vi "UHR-Fleezers Control (fpga) - avogadro 6 - symmetric position FB_raster scan ALEX.vi"() -> ()   [LabVIEW 2014]
doc: "UHR-Fleezers Instrument Control Code (fpga)"
uses:
  <vilib>/Platform/TimedLoop/XDataNode/timing_clust.ctl
  <vilib>/Platform/TimedLoop/XDataNode/nitl_modes.ctl
  <vilib>/Platform/TimedLoop/XDataNode/wakeup.ctl
  <vilib>/rvi/Emulation/niFpgaGetClockAttributes.vi
  <vilib>/rvi/Emulation/niFpgaSctlEmulationGetInTimedLoop.vi
  <vilib>/rvi/Emulation/niFpgaEmulationReportErrorSimple.vi
  <vilib>/rvi/Emulation/niFpgaProcessEmulError.vi
  <vilib>/rvi/eio/common/nirviEmuTemplateMethod_errors.vi
  <vilib>/rvi/interface/RandomDataEmulation/niFpgaRandomDataHandleErrors.vi
  <vilib>/rvi/Emulation/niFpgaCriticalErrorInLSC.vi
  <vilib>/rvi/Emulation/niFpgaEmulationIsFPGAContextNoSignature.vi
  <vilib>/rvi/errors/niFpgaSetErrorForExecOnDevCompSimple.vi
  <vilib>/rvi/eio/common/nirviEmuReportErrorAndStop.vi
  <vilib>/rvi/DataTransferAndStorage/Container/Common/niFpgaContainerGetUniqueNameForEmu.vi
  <vilib>/rvi/FIFO/Fifo_Resource/nirvififoEmulationSetSize.vi
  <vilib>/rvi/FIFO/Fifo_Resource/nirviFifoEmulationQueueMgr.vi
  <instcachedir>/0/nirviFifoEmulationQueueMgr_E5CAEC123FF24DC58D834DCA3CDAA9B5.lvgen/nirviFifoEmulationQueueMgr_E5CAEC123FF24DC58D834DCA3CDAA9B5_001.vi
  <vilib>/rvi/FIFO/Fifo_Resource/nirvififoEmulationDetermineInputValidOut.vi
  <vilib>/rvi/FIFO/Fifo_Resource/nirvififoEmulationCreateLock.vi
  <vilib>/rvi/FIFO/Fifo_Resource/nirvififoEmulationObtainLock.vi
  <vilib>/rvi/FIFO/Fifo_Resource/nirvififoEmulationReleaseLock.vi
  <vilib>/rvi/occurrence/nirviWaitOnOccurrenceBase.vi
  <vilib>/rvi/errors/nirviReportUnexpectedCaseInternalError.vi
  <vilib>/rvi/errors/nirviReportUnexpectedCaseInternalError (U32).vi
  <vilib>/rvi/DataTransferAndStorage/Container/Common/niFpgaContainerExecOnDevCompGetState.vi
  <vilib>/Utility/error.llb/Clear Errors.vi
  <vilib>/eio/EIONode/EIONode.xnode
  <vilib>/eio/EIOMethodNode/EIOMethodNode.xnode
  <vilib>/rvi/DataTransferAndStorage/Container/XNode/niFpgaContainer.xnode
  <vilib>/rvi/interface/RandomDataEmulation/nirviRandomDataFpgaReadWriteTemplate.vi
  <vilib>/rvi/FIFO/Fifo_Resource/nirvififoEmulationWrite.vi
  <vilib>/rvi/FIFO/Fifo_Resource/niFpgaFifoEmulationRefIn.vi
  <vilib>/addons/control/pid/fpga.llb/XNode/niFpgaPID.xnode
  <vilib>/Platform/TimedLoop/XDataNode/XDataNode.xnode
  <vilib>/rvi/FIFO/Fifo_Resource/nirvififoEmulationRead.vi
  <vilib>/Platform/TimedLoop/XDataNode/XDNodeRunTimeDep.lvlib
  <vilib>/rvi/Memory/Memory_Emulation/niFpgaMemoryEmulationRefIn.vi
panel:
  in  "BD 1 Delay (ticks)":u8
  out "lifetime (ticks)":u16
  in  "Lifetime to FIFO":bool
  in  "Tab Control":T1(tab)=enum."MCL trap control"
  in  "Set 3":bool
  in  "Set 2":bool=TRUE
  in  "Set 1":bool=TRUE
  in  "Trap Pos to FIFO":bool
  in  "N of AI1 Int Acq Sets":i16=2 min=1 max=3 step=1
  out "AI Late Counter":u8
  in  "ai count":u16=400
  in  "+ phase":bool
  in  "Phase count adjustment":i16
  out "Relative phase":i16
  in  "AI to FIFO":bool
  out "BD1 Frequency Out 1":u64
  out "BD1 Frequency Out 2":u64
  out "Trap Pos FIFO Timeout":u16
  out "Trap AI FIFO Timeout":u16
  in  "Trap FIFO Set Timeout":i32
  in  "Tab Control 2":T2(tab)
  in  "Multiple trap 3 position offset \nfile":bool
  in  "Piezo offset Y points":u64
  in  "Piezo offset X points":u64
  in  "Piezo offset Xmin":u64
  in  "Piezo Offset Ymin":u64
  in  "Piezo Offset Increment":u64
  out "BD1 amplitude 1 out":u16
  out "BD1 amplitude 2 out":u16
  in  "FB output range":cluster{"output low":i16, "output high":i16}={"output low"=0, "output high"=3000}
  in  "FB Gains":T3={"proportional gain (Kc)"=10, "integral gain (Kc*Ts/Ti)"=5, "derivative gain (Kc*Td/Ts)"=0}
  in  "RF synth green feedback max":i16=4000
  in  "RD":bool=TRUE
  in  "Swap F1 and F2":bool
  in  "Cont. Scan":bool
  in  "Abort scan":bool
  in  "Cycles per step":u64
  in  "Scan BD":bool
  in  "Number of scans":u16
  in  "Scan steps":u64
  in  "Scan freq.  increment":i64
  out "Scanning":bool
  in  "Start scan":bool
  in  "OSK Bd 1":bool
  in  "Reset Bd 1":bool
  in  "PMODE":bool=TRUE
  in  "Number Interlace Cycles":u8=2 min=1 max=3
  in  "Interlace Off Parameters":u8=1 min=1 max=3
  in  "Interlace ON/OFF":bool
  out "DIO Relative phase":i16
  in  "Phase count adjustment (DIO)":i16
  in  "+ phase (DIO)":bool
  out "DIO Late Counter":u8
  in  "DIO count 1 (ticks)":u16=400
  in  "DIO count 2 (ticks)":u16=400
  in  "DIO count 3 (ticks)":u16=400
  out "AI2 Y Sum Set 2":i16
  out "AI2 Y Sum Set 1":i16
  in  "FB Setpoint Set 1":i16 min=0 step=1
  in  "FB Reset Set 1":bool
  in  "FB On/Off Set 1":bool
  in  "FB Reset Set 2":bool
  in  "FB On/Off Set 2":bool
  in  "FB Setpoint Set 2":i16 min=0 step=1
  out "Scan I":u64
  in  "Amp switch delay":u8=5
  in  "RF synth bd controls green":bool
  in  "Phase Trap 2":fxp<+,14,14>
  in  "Phase Trap 1":fxp<+,14,14>
  in  "Phase offset method":u8
  in  "BD 2 Amplitude 1":u16
  in  "BD 1 Amplitude 1":u16
  in  "BD 2 Frequency 1":u64
  in  "BD 1 Frequency 1":u64
  in  "BD 2 Amplitude 2":u16
  in  "BD 1 Amplitude 2":u16
  in  "BD 2 Frequency 2":u64
  in  "BD 1 Frequency 2":u64
  in  "BD 2 Amplitude 3":u16
  in  "BD 1 Amplitude 3":u16
  in  "BD 2 Frequency 3":u64
  in  "BD 1 Frequency 3":u64
  in  "BD 2 Delay (Ticks)":u8 caption="Count(Ticks)"
  in  "Next trap write delay (ticks)":u8 caption="Count(Ticks)"
  out "Random phase generated":fxp<+,14,14>
  in  "RF phase reset before cycles":bool
  in  "Trap 1 osc enable":bool
  in  "N trap osc periods":i16
  in  "Trap osc period (pts)":i16
  in  "Osc traps":bool
  in  "Initiate trap osc":bool
  in  "Ready Write":bool
  in  "Data":i64
  in  "Address 2":u32
  in  "Osc trap cont.":bool
  in  "Trap 2 osc enable":bool
  out "Piezo X out":i16
  out "Piezo Y out":i16
  in  "Piezo Trap ON/Off (AO3)":i16
  in  "Piezo Trap X (AO5)":i16
  in  "Piezo Trap Y (AO4)":i16
  in  "Symmetric force feedback\nand raster scan":bool
  in  "FB Min frequency":u64
  in  "FB Max Frequency":u64
  in  "Dynamic Force FB (Ronen)":bool
  in  "Trap pos. FB Range":T4={"FB2 output low"=-1.0, "FB2 output high"=0.999969482421875}
  in  "Trap Pos. FB Gains":T5={"proportional gain (Kc)"=0.999969482421875, "integral gain (Kc*Ts/Ti)"=0.999969482421875, "derivative gain (Kc*Td/Ts)"=0.0}
  in  "B factor":fxp<+/-,32,16>
  in  "Negate Diff?":bool
  in  "Diff FB Measurement?":bool
  in  "FB Trig Integrate":u32=1
  out "TTrig?":bool
  in  "TTrig Negate Pos":bool=TRUE
  out "Trap Pos FB Int Signal":fxp<+/-,24,9> format="%.18g"
  out "Trap Pos FB Int-Norm Signal":fxp<+/-,16,1> format="%.16g"
  in  "FPGA TTrig Thresh":i64
  in  "FPGA Trap Trig":bool
  out "Trap Pos FB Action":i64
  in  "Trap Pos. FB Offset Factor":i64
  in  "Trap Pos. FB Mult Factor":i64=2
  in  "Trap Pos. FB Reset":bool
  in  "Trap Pos FB Monitor T1 or T2":bool
  in  "AI1 X Scale":u16
  in  "Trap Pos FB Int Count":u16=100
  in  "Trap Pos FB Negate Action":bool
  out "AI1 X Set 2":fxp<+/-,16,1>
  out "AI1 X Set 1":fxp<+/-,16,1>
  in  "Trap Pos. FB SP":fxp<+/-,16,1>
  in  "Force feedback":bool
  out "TTrig Sig":i64
  out "TTrig Fin Thresh":i64
  in  "ScanTrap 3 or Fl-laser":bool
  in  "1D or 2D Scan?":bool
  in  "Abort scan (MCL)":bool
  in  "MCL Scan Axis":bool
  in  "Cont. Scan (MCL)":bool
  out "Scan I (MCL)":u64
  in  "Number of scans (MCL)":u16
  out "Scanning MCL":bool
  in  "Scan steps (MCL)":u64
  in  "Cycles per step (MCL)":u64
  in  "Scan freq.  increment (MCL)":i16
  in  "Start scan (MCL)":bool
  in  "AO2 (X)":i16
  in  "AO1 (Y)":i16
  out "MCL Late Counter":u8
  in  "MCL count":u32=800
  out "MCL Relative Phase":i16
  in  "Phase count adjustment (MCL)":i16
  in  "+ phase (MCL)":bool
  in  "Lifetime events to read blue":u16=100
  in  "Lifetime read blue fifo":bool
  out "lifetime events in fifo":u16
  out "APD2 int gate":bool
  out "APD3 out state":bool
  in  "APD Gate Operating Mode":u8 max=2 step=1
  in  "Invert APD Gate":bool
  in  "APD Gate OFF Count":u16=100
  in  "APD Gate ON Count":u16=300
  out "APD 1 Gate Late Counter":u8
  out "APD 1 Gate Relative Phase":i16
  in  "Phase count adjustment (APD 1 Gate)":i16
  in  "+ phase (APD 1 Gate)":bool
  out "APD 2 Counts 0":u32
  out "APD 2 Counts 1":u32
  out "APD 1 Counts 0":u32
  out "APD 1 Counts 1":u32
  out "APD1 out state":bool
  in  "APD AO scale factor":i16=1
  in  "APD to FIFO":bool
  in  "APD Acq Rate Count":u32=20000000
  out "APD Acq Late Counter":u8
  out "APD Acq Relative Phase":i16
  in  "Phase Count Adjustment (APD Acq)":i16
  in  "+ phase (APD Acq)":bool
  in  "Phase count adjustment (APD 2 Gate)":i16
  out "APD 2 Gate Late Counter":u8
  out "APD 2 Gate Relative Phase":i16
  in  "+ phase (APD 2 Gate)":bool
  out "APD2 out state":bool
  out "APD 3 Counts 0":u32
  out "APD 3 Counts 1":u32
  out "APD 3 Gate Late Counter":u8
  in  "Phase count adjustment (APD 3 Gate)":i16
  out "APD 3 Gate Relative Phase":i16
  in  "+ phase (APD 3 Gate)":bool
  out "APD1 int gate":bool
  out "APD3 int gate":bool
  in  "Lifetime timeout APD1":u16=200
  in  "Laser choice 2":u8=100
  in  "Laser choice 1":u8=100
  in  "Laser choice 0":u8=100
  in  "FL interlace OFF count 2":u16=100
  in  "FL interlace OFF count 1":u16=100
  in  "FL interlace ON count 2":u16=300
  in  "Fl interlace ON count 1":u16=300
  in  "D3 2":i16
  in  "I3 2":i16=5
  in  "P3 2":i16=10
  in  "Green FB Setpoint 2":i16=250 min=0 step=1
  in  "Green FB Reset 2":bool
  in  "D3":i16
  in  "I3":i16=5
  in  "P3":i16=10
  in  "Green Filter Flipper":bool
  in  "Green FB Count":u16=1200
  out "Green Late Counter":u8
  out "Green FB Relative Phase":i16
  in  "Phase count adjustment (Green FB)":i16=10
  in  "+ phase (Green FB)":bool
  out "Green FB Sum":i16
  in  "Green int current ON count adj":u16=150
  in  "Current Out":u16=30000
  in  "Green FB On/Off":bool
  in  "Green FB Setpoint":i16=250 min=0 step=1
  in  "Green FB Reset":bool
  in  "Operating Mode 2":u8=2 max=2 step=1
  in  "Invert GI 2":bool
  in  "Green interlace OFF count 2":u16=900
  in  "Green interlace ON count 2":u16=300
  out "GI Late Counter 2":u8
  out "GI Relative phase 2":i16
  in  "Phase count adjustment (GI) 2":i16=20
  in  "+ phase (GI) 2":bool
  in  "FL interlace OFF count 0":u16=100
  out "GI Relative phase":i16
  in  "Phase count adjustment (GI)":i16
  in  "+ phase (GI)":bool
  in  "FL interlace ON count 0":u16=300
  out "GI Late Counter":u8
  in  "Invert GI":bool
  in  "Operating Mode":u8 max=2 step=1
  out "green FB running":bool
  in  "+ phase (RI)":bool
  out "RI Relative phase":i16
  out "RI Late Counter":u8
  in  "Red interlace ON count":u16=300
  in  "Red interlace OFF count":u16=100
  in  "Invert RI":bool
  in  "Red Laser Operating Mode":u8 max=2 step=1
  in  "Phase count adjustment (RI)":i16
  out "Red FB Intensity":i16
  in  "RI Current Out":u16=30000
  in  "Red FB On/Off":bool
  in  "D4":i16
  in  "I4":i16=5
  in  "P4":i16=10
  in  "Red FB Setpoint":i16=250 min=0 step=1
  in  "Red FB Reset":bool
  in  "RI Operating Mode 2":u8=2 max=2 step=1
  in  "Invert RI 2":bool
  in  "Phase count adjustment (BI AO)":i16=20
  in  "Blue current ON count adj (AO)":u16=150
  in  "BI Current Out":i16=30000
  in  "Blue FB On/Off":bool
  in  "D5":i16
  in  "I5":i16=5
  in  "P5":i16=10
  in  "Blue FB Setpoint":i16=250 min=0 step=1
  in  "Blue FB Reset":bool
  in  "BI Operating Mode (AO)":u8=2 max=2 step=1
  in  "Invert BI (AO)":bool
  in  "Blue OFF count (AO)":u16=900
  in  "Blue ON count (AO)":u16=300
  out "BI Late Counter (AO)":u8
  out "BI Relative phase (AO)":i16
  in  "+ phase (BI AO)":bool
  in  "Phase count adjustment (BI D)":i16
  in  "Blue Laser Operating Mode (D)":u8 max=2 step=1
  in  "Invert BI (D)":bool
  in  "Blue interlace OFF count (D)":u16=100
  in  "Blue interlace ON count (D)":u16=300
  out "Blue Late Counter (D)":u8
  out "BI Relative phase (D)":i16
  in  "+ phase (BI D)":bool
  out "Blue Intensity":i16
  in  "Invert EMCCD Gate":bool
  in  "EMCCD Gate ON count":u16=300
  in  "EMCCD Gate OFF count":u16=100
  out "EMCCD Late counter":u8
  out "EMCCD relative phase":i16
  in  "+ phase (EMCCD Gate)":bool
  in  "EMCCD Gate Operating Mode":u8 max=2 step=1
  in  "Phase Count Adjustment EMCCD Gate":i16
  # "Raster Scan AOD"
  # "1 (X)"
  # "2 (Y)"
  # "IR Intensity Feedback (RF BD 1)"
  # "FB Gains Set 1"
  # "FB output range 1"
  # "IR Intensity Feedback (RF BD 2) -\nonly when using BD 2 for green laser AOM (not trap Y)"
  # "Keep below 4096 (12 bits) to stay within range of RF board. Going over doesn't saturate, it truncates higher bits."
  # "RF phase offset control"
  # "Methods are:\n0 - Default, do nothing at all (no phase offset writes)\n1 - Manual phase adjustment\n2 - Cycle the phase adjustment using the input phase numbers as increment values for each cycle"
  # "False is usual, True is external loop method"
  # "Parameters if using the external RF switching loop"
  # "Parameters if using the usual internal RF switching method"
  # "FB Triggering Excitation Laser"
  # "Trap Pos. FB Gains"
  # "Trap Pos. FB Range"
  # "AO1 (Y)"
  # "2D"
  # "Trap 3"
  # "1D"
  # "AO2 (X)"
  # "Fl Laser"
  # "APD AO for aligning"
  # "Detection Loop"
  # "Green fluorescent laser digital gate interlacing loop"
  # "0 Forced ON\n1 Forced OFF\n2 Interlacing"
  # "ALEX settings:"
  # "Controls for usual IA ME controls green AOM"
  # "Controls for RF synth board controls green AOM"
  # "Green FB Gains"
  # "Red fluorescent laser digital gate interlacing loop"
  # "Detection Loop"
  # "0 Forced ON\n1 Forced OFF\n2 Interlacing"
  # "Analog/FB Control Loop\n(Disabled)"
  # "Digital Control Loop"
  # "Blue laser intensity reading"
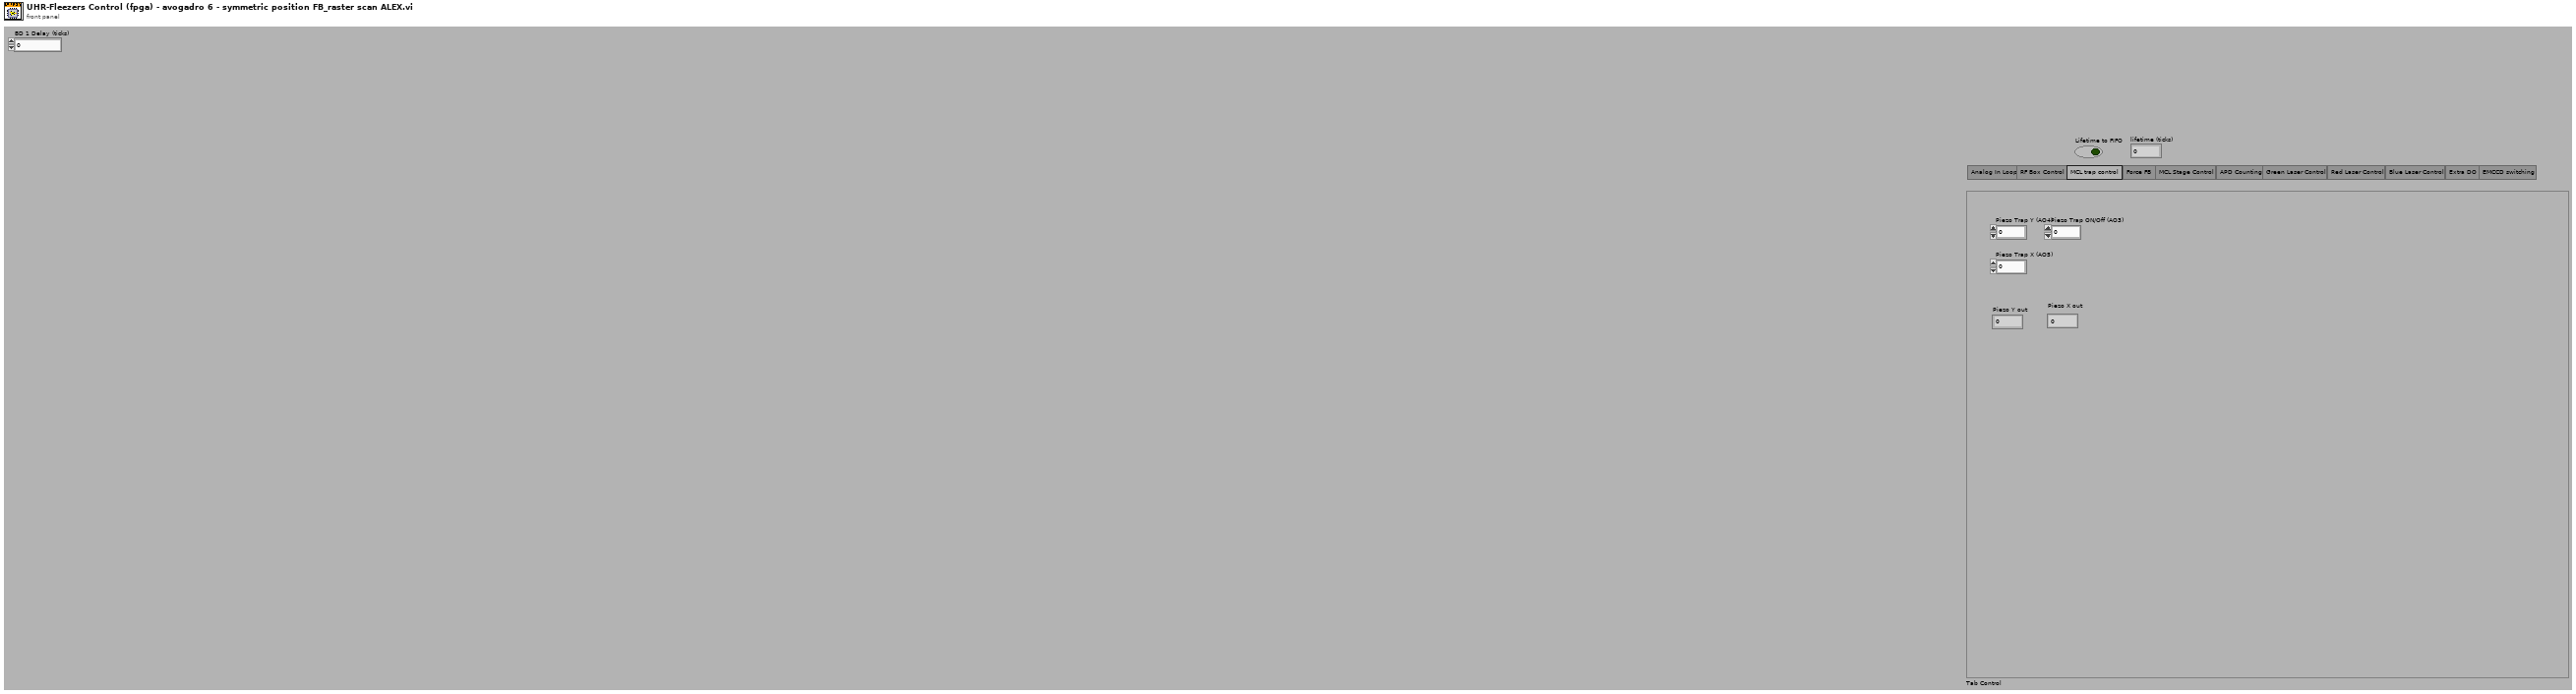
[diagram p1: front panel]
types:
  T1 = enum32{"Analog In Loop", "RF Box Control", "MCL trap control", "Force FB", "MCL Stage Control", "APD Counting", "Green Laser Control", "Red Laser Control", "Blue Laser Control", "Extra DO", "EMCCD switching"}
  T2 = enum32{"Controls", "Interlacing Frequency and Amplitude Values", "Oscillate trap from memory"}
  T3 = cluster{"proportional gain (Kc)":i16, "integral gain (Kc*Ts/Ti)":i16, "derivative gain (Kc*Td/Ts)":i16}
  T4 = cluster{"FB2 output low":fxp<+/-,16,1>, "FB2 output high":fxp<+/-,16,1>}
  T5 = cluster{"proportional gain (Kc)":fxp<+/-,16,1>, "integral gain (Kc*Ts/Ti)":fxp<+/-,16,1>, "derivative gain (Kc*Td/Ts)":fxp<+/-,16,1>}
  T6 = typedef "XDNodeRunTimeDep.lvlib/timing_clust.ctl" = cluster{"Expected End [f-1]":u64, "Actual End [f-1]":u64, "Finished Late? [f-1]":bool, "Expected End [i-1]":u64, "Actual End [i-1]":u64, "Finished Late? [i-1]":bool, "Expected Start [i]":u64, "Actual Start [i]":u64, "Expected Start [f]":u64, "Actual Start [f]":u64, "Source Name":string, "Structure Name":string, "Period":i64, "Deadline":i64, "Offset":i64, "Start":i64, "Priority":i32, "Timeout":i32, "Mode":T7, "Wakeup Reason":T8, "Error":errorcluster, "Source Type":string, "Secondary Source Type":string, "Global End Time":u64, "Global Start Time":u64, "Frame Duration":u64, "Iteration Duration":u64, "Assigned CPU":i32, "I/O Scan Engine Mode":u32}
  T7 = typedef "XDNodeRunTimeDep.lvlib/nitl_modes.ctl" = enum32{"No Change", "Process missed periods, maintain original phase", "Discard missed periods, maintain original phase", "Process missed periods, ignore original phase", "Discard missed periods, ignore original phase"}
  T8 = typedef "XDNodeRunTimeDep.lvlib/wakeup.ctl" = enum32{"Normal", "Aborted", "Asynchronous wakeup", "Timing source error", "Timed loop error", "Timeout"}
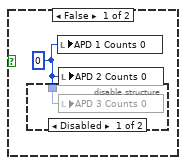
[diagram p4: hidden frame]
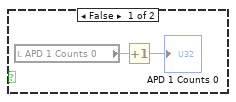
[diagram p9: hidden frame]
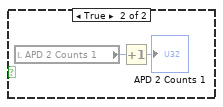
[diagram p11: hidden frame]
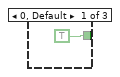
[diagram p13: hidden frame]
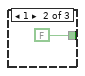
[diagram p14: hidden frame]
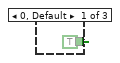
[diagram p15: hidden frame]
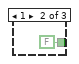
[diagram p16: hidden frame]
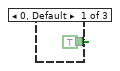
[diagram p18: hidden frame]
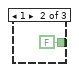
[diagram p19: hidden frame]
diagram:
  w11 = i16 0
  w15 = FALSE
  # "EMCCD gating"
  # "BD2 amp"
  # "BD1 amp"
  # "BD2 amp"
  # "BD1 amp"
  # "timing array current index"
  # "timing array"
  # "timing counter (phase adjusted here)"
  # "late counter"
  n1 = disable-structure shown="Disabled" {
    frame Disabled {
      w16 = i16 2 items=["UnSet Ready", "ReadWrite", "Wait Ready"]
      n2 = while "Handshake memory transfer for trap oscillation sin wave data" {
        shift-right: [w18] -> _
        shift-left: w16 -> [w19]
        stop <- FALSE stop-if-true
        # "Write"
        n3 = case shown="1" w19 {
          tunnel: [w22 w27 w28] -> w18
          frame 3, Default {
            w20 = i16 2 items=["UnSet Ready", "ReadWrite", "Wait Ready"]
            w21 = i16 1 items=["UnSet Ready", "ReadWrite", "Wait Ready"]
            n4 = Select(t=w21, s="Ready Write", f=w20) -> (s? t:f=w22:i16)
          }
          frame 1 {
            w27 = i16 0 items=["UnSet Ready", "ReadWrite", "Wait Ready"]
            n5 = xnode ("Memory Write")("Address"="Address 2", "Data"="Data", "Memory In"=refnum<k21> "Trap osc memory") -> ()  [unwired: 1 out]
          }
          frame 0 {
            w28 = i16 2 items=["UnSet Ready", "ReadWrite", "Wait Ready"]
            n6 = local write "Ready Write"(FALSE ("Ready Read")) -> ()
          }
        }
      }
    }
    frame Enabled {
    }
  }
  n7 = flat-sequence "FPGA initialization to do before running any of the loops" {
    tunnel: [u16 0 ("DIO count 3 (ticks)")] -> w4
    tunnel: [w37] -> _
    frame #0 {
      # "UDCLK out enable and set low"
      # "WR"
      # "BD 2"
      # "BD 1"
      # "With the RF synth board initialization now done in a separate fpga vi, now when this vi is started, board is already configured and is ready for interlacing. Just need to set WR high and enabled UDCLK as write and set to low.\nbefore setting data and address bits."
      # "Start up expansion chassis early\nto avoid delays later"
      # "Set data and address values to something safe (a correct setting) so any initial WR and udclk flipping doesn't have a chance to mess anything up. Safe would be setting an unused data entry:"
      n8 = xnode "FPGA I/O Method Node"("Enable"=TRUE) -> ("FPGA I/O Out"=w31:refnum<k21>)  [unwired: 1 in]
      n9 = xnode "FPGA I/O Method Node"("Enable"=TRUE) -> ("FPGA I/O Out"=w34:refnum<k21>)  [unwired: 1 in]
      n10 = xnode "FPGA I/O Node"("Chassis2/Mod1/AO0"=u16 0 ("Chassis2/Mod4/AO0")) -> ("Chassis2/Mod2/AI0"=w37:i16)  [unwired: 2 in, 2 out]
      n11 = xnode "FPGA I/O Node"("Connector1/DIO15"=TRUE) -> ()  [unwired: 1 in, 1 out]
      n12 = xnode "FPGA I/O Node"("I/O Item"=FALSE ("Connector1/DIO30"), "FPGA I/O In"=w31) -> ()  [unwired: 1 out]
      n13 = xnode "FPGA I/O Node"("I/O Item"=FALSE ("Connector1/DIO30"), "FPGA I/O In"=w34) -> ()  [unwired: 1 out]
      n14 = xnode "FPGA I/O Node"("Connector1/DIO0"=FALSE, "Connector1/DIO1"=FALSE, "Connector1/DIO2"=FALSE, "Connector1/DIO3"=FALSE, "Connector1/DIO4"=FALSE, "Connector1/DIO5"=FALSE, "Connector1/DIO6"=FALSE, "Connector1/DIO7"=FALSE, "Connector1/DIO8"=FALSE, "Connector1/DIO9"=FALSE, "Connector1/DIO10"=FALSE, "Connector1/DIO11"=FALSE, "Connector1/DIO12"=FALSE, "Connector1/DIO13"=FALSE, "Connector1/DIO20"=FALSE, "Connector1/DIO21"=FALSE, "Connector1/DIO22"=FALSE, "Connector1/DIO23"=FALSE, "Connector1/DIO24"=FALSE, "Connector1/DIO25"=FALSE, "Connector1/DIO26"=FALSE, "Connector1/DIO27"=FALSE, "Connector1/DIO14"=FALSE) -> ()  [unwired: 23 in, 23 out]
    }
  }
  n15 = node-c288() -> (w7:T6)  [unwired: 1 in]
  n16 = timed-loop "RF box board DIO control: control bits" {
    timing: w7 -> [_]
    timing-out: [_] -> w6
    tunnel: [w65] -> _
    tunnel: w4 -> [w65]
    stop <- FALSE stop-if-true
    n17 = xnode "FPGA I/O Node"("Connector1/DIO16"="RD", "Connector1/DIO17"="PMODE", "Connector1/DIO18"="OSK Bd 1", "Connector1/DIO19"="Reset Bd 1", "Connector0/DIO3"="Green Filter Flipper") -> ()  [unwired: 5 in, 5 out]
  }
  n18 = node-c288(w6) -> ()
  n19 = local read "AO1 (Y)"() -> (w13:i16)
  n20 = local read "AO2 (X)"() -> (w12:i16)
  n21 = To Unsigned Long Integer(number=w4) -> (unsigned 32bit integer=w3:u32)
  n22 = disable-structure shown="Disabled" {
    disable-tunnel: w4 -> [w73 _]
    disable-tunnel: [w72 _] -> w5
    frame Disabled {
      w72 = FALSE
      n23 = while "APD 1 Gating" {
        shift-right: [w128] -> _
        shift-left: w73 -> [w133]
        shift-right: [w127] -> _
        shift-left: w72 -> [w125]
        stop <- FALSE stop-if-true
        n24 = flat-sequence {
          tunnel: w133 -> [w136]
          tunnel: [w137] -> w131
          tunnel: [w136] -> w129
          tunnel: [w135] -> w126
          tunnel: w125 -> [w135]
          tunnel: [w140] -> w132
          tunnel: w131 -> [w140]
          tunnel: [w139] -> w130
          tunnel: w129 -> [w139]
          tunnel: w126 -> [w138]
          tunnel: [w158] -> w128
          tunnel: w132 -> [w172]
          tunnel: w130 -> [w169]
          tunnel: [w141] -> w127
          frame #0 {
            n25 = call "Loop Timer7"("Count(Ticks)"=w136) -> ("Tick Count(Ticks)"=w137:u16)
          }
          frame #1 {
            # "Signal maybe then sent through \na transistor before APD"
            n26 = xnode "FPGA I/O Node"("Connector0/DIO0"=w138) -> ()  [unwired: 1 in, 1 out]
            "APD1 int gate" <- w138
          }
          frame #2 {
            n27 = feedback #1(TRUE) -> (w164:bool)
            n28 = feedback-in #2(w172) -> ()
            n29 = feedback #2(w172) -> (w171:u16)
            n30 = Not(x=w164) -> (.not. x?=w161:bool)
            n31 = feedback-in #1(w161) -> ()
            n32 = Subtract(x=w172, y=w171) -> (x-y=w170:u16)
            n33 = Select(t="APD Gate ON Count", s=w161, f="APD Gate OFF Count") -> (s? t:f=w166:u16)
            n34 = Subtract(x=w170, y=w169) -> (x-y=w146:u16)
            n35 = Subtract(x=w166, y=w146) -> (x-y=w157:u16)
            n36 = Number To Boolean Array(number=w146) -> (Boolean array=w147:bool[])
            n37 = Or Array Elements(Boolean array=w147) -> (logical OR=w145:bool)
            n38 = Boolean To (0,1)(Boolean="+ phase (APD 1 Gate)") -> (0, 1=w155:i16)
            n39 = Boolean To (0,1)(Boolean=w145) -> (0, 1=w152:i16)
            n40 = Multiply(x=w155, y="Phase count adjustment (APD 1 Gate)") -> (x*y=w153:i16)
            n41 = To Unsigned Byte Integer(number=w152) -> (unsigned 8bit integer=w149:u8)
            n42 = Add(x=w157, y=w153) -> (x+y=w158:u16)
            n43 = feedback #3(i16 0) -> (w160:i16)
            n44 = Subtract(x=w160, y=w153) -> (x-y=w159:i16)
            "APD 1 Gate Relative Phase" <- w159
            n45 = feedback-in #3(w159) -> ()
            n46 = feedback #4(u8 0) -> (w150:u8)
            n47 = Add(x=w149, y=w150) -> (x+y=w148:u8)
            "APD 1 Gate Late Counter" <- w148
            n48 = feedback-in #4(w148) -> ()
            n49 = case shown="2" "APD Gate Operating Mode" {
              tunnel: [TRUE FALSE w175] -> w142
              tunnel: w164 -> [_ _ w175]
              frame 0, Default {
              }
              frame 1 {
              }
              frame 2 {
              }
            }
            n50 = Not(x=w142) -> (.not. x?=w143:bool)
            n51 = Select(t=w143, s="Invert APD Gate", f=w142) -> (s? t:f=w141:bool)
          }
        }
      }
      n52 = while "APD 2 Gating" {
        shift-right: [w77] -> _
        shift-left: w73 -> [w82]
        shift-right: [w76] -> _
        shift-left: w72 -> [w74]
        stop <- FALSE stop-if-true
        n53 = flat-sequence {
          tunnel: w82 -> [w85]
          tunnel: [w86] -> w80
          tunnel: [w85] -> w78
          tunnel: [w84] -> w75
          tunnel: w74 -> [w84]
          tunnel: [w89] -> w81
          tunnel: w80 -> [w89]
          tunnel: [w88] -> w79
          tunnel: w78 -> [w88]
          tunnel: w75 -> [w87]
          tunnel: [w111] -> w77
          tunnel: w81 -> [w121]
          tunnel: w79 -> [w119]
          tunnel: [w90] -> w76
          frame #0 {
            n54 = call "Loop Timer8"("Count(Ticks)"=w85) -> ("Tick Count(Ticks)"=w86:u16)
          }
          frame #1 {
            # "Signal maybe then sent through \na transistor before APD"
            n55 = xnode "FPGA I/O Node"("Connector0/DIO1"=w87) -> ()  [unwired: 1 in, 1 out]
            "APD2 int gate" <- w87
          }
          frame #2 {
            n56 = local read "APD Gate ON Count"() -> (w104:u16)
            n57 = local read "APD Gate OFF Count"() -> (w103:u16)
            n58 = feedback #5(TRUE) -> (w116:bool)
            n59 = feedback-in #6(w121) -> ()
            n60 = feedback #6(w121) -> (w105:u16)
            n61 = Not(x=w116) -> (.not. x?=w114:bool)
            n62 = feedback-in #5(w114) -> ()
            n63 = Subtract(x=w121, y=w105) -> (x-y=w120:u16)
            n64 = Select(t=w104, s=w114, f=w103) -> (s? t:f=w118:u16)
            n65 = Subtract(x=w120, y=w119) -> (x-y=w96:u16)
            n66 = Subtract(x=w118, y=w96) -> (x-y=w110:u16)
            n67 = Number To Boolean Array(number=w96) -> (Boolean array=w95:bool[])
            n68 = Or Array Elements(Boolean array=w95) -> (logical OR=w94:bool)
            n69 = Boolean To (0,1)(Boolean="+ phase (APD 2 Gate)") -> (0, 1=w108:i16)
            n70 = Multiply(x=w108, y="Phase count adjustment (APD 2 Gate)") -> (x*y=w106:i16)
            n71 = Boolean To (0,1)(Boolean=w94) -> (0, 1=w101:i16)
            n72 = Add(x=w110, y=w106) -> (x+y=w111:u16)
            n73 = To Unsigned Byte Integer(number=w101) -> (unsigned 8bit integer=w98:u8)
            n74 = feedback #7(i16 0) -> (w113:i16)
            n75 = Subtract(x=w113, y=w106) -> (x-y=w112:i16)
            "APD 2 Gate Relative Phase" <- w112
            n76 = feedback-in #7(w112) -> ()
            n77 = feedback #8(u8 0) -> (w99:u8)
            n78 = Add(x=w98, y=w99) -> (x+y=w97:u8)
            "APD 2 Gate Late Counter" <- w97
            n79 = feedback-in #8(w97) -> ()
            n80 = local read "APD Gate Operating Mode"() -> (w102:u8)
            n81 = case shown="2" w102 {
              tunnel: [TRUE FALSE w124] -> w91
              tunnel: w116 -> [_ _ w124]
              frame 0, Default {
              }
              frame 1 {
              }
              frame 2 {
              }
            }
            n82 = local read "Invert APD Gate"() -> (w93:bool)
            n83 = Not(x=w91) -> (.not. x?=w92:bool)
            n84 = Select(t=w92, s=w93, f=w91) -> (s? t:f=w90:bool)
          }
        }
      }
    }
    frame Enabled {
    }
  }
  n85 = disable-structure shown="Disabled" {
    disable-tunnel: w4 -> [w176 _]
    frame Disabled {
      n86 = while "Excitation laser intensity feedback measurement (all lasers)" {
        shift-right: [w177] -> _
        shift-left: w176 -> [w182]
        stop <- FALSE stop-if-true
        n87 = flat-sequence {
          tunnel: w182 -> [w184]
          tunnel: [w185] -> w180
          tunnel: [w184] -> w178
          tunnel: [w191] -> w181
          tunnel: w180 -> [w191]
          tunnel: [w190] -> w179
          tunnel: w178 -> [w190]
          tunnel: [w203] -> w177
          tunnel: w181 -> [w214]
          tunnel: w179 -> [w211]
          frame #0 {
            n88 = call "Loop Timer9"("Count(Ticks)"=w184) -> ("Tick Count(Ticks)"=w185:u16)
          }
          frame #1 {
            # "Design note:\n\nAll lasers need to be measured at the same \ntime because the AI expansion module\ncannot independently time the measurements\nwithin our requirements: there is dead time.\n\nThis probably wouldn't be an issue with the built\nin AI on the fpga board itself."
            n89 = xnode "FPGA I/O Node"("Connector1/DIO35"=TRUE) -> ("Chassis2/Mod1/AI2"=→"Blue Intensity", "Chassis2/Mod1/AI1"=→"Red FB Intensity", "Chassis2/Mod1/AI0"=→"Green FB Sum")  [unwired: 4 in, 4 out]
          }
          frame #2 {
            n90 = feedback-in #9(w214) -> ()
            n91 = feedback #9(w214) -> (w213:u16)
            n92 = Subtract(x=w214, y=w213) -> (x-y=w212:u16)
            n93 = xnode "FPGA I/O Node"("Connector1/DIO35"=FALSE) -> ()  [unwired: 1 in, 1 out]
            n94 = Subtract(x=w212, y=w211) -> (x-y=w193:u16)
            n95 = Subtract(x="Green FB Count", y=w193) -> (x-y=w207:u16)
            n96 = Number To Boolean Array(number=w193) -> (Boolean array=w194:bool[])
            n97 = Or Array Elements(Boolean array=w194) -> (logical OR=w192:bool)
            n98 = Boolean To (0,1)(Boolean="+ phase (Green FB)") -> (0, 1=w205:i16)
            n99 = Boolean To (0,1)(Boolean=w192) -> (0, 1=w199:i16)
            n100 = Multiply(x=w205, y="Phase count adjustment (Green FB)") -> (x*y=w200:i16)
            n101 = Add(x=w207, y=w200) -> (x+y=w203:u16)
            n102 = To Unsigned Byte Integer(number=w199) -> (unsigned 8bit integer=w196:u8)
            n103 = feedback #10(i16 0) -> (w202:i16)
            n104 = Subtract(x=w202, y=w200) -> (x-y=w201:i16)
            "Green FB Relative Phase" <- w201
            n105 = feedback-in #10(w201) -> ()
            n106 = feedback #11(u8 0) -> (w197:u8)
            n107 = Add(x=w196, y=w197) -> (x+y=w195:u8)
            "Green Late Counter" <- w195
            n108 = feedback-in #11(w195) -> ()
          }
        }
      }
    }
    frame Enabled {
    }
  }
  n109 = disable-structure shown="Disabled" {
    disable-tunnel: w4 -> [w215 _]
    frame Disabled {
      n110 = while "APD 2 Counter" {
        tunnel: w215 -> [_]
        stop <- FALSE stop-if-true
        n111 = flat-sequence {
          frame #0 {
            n112 = xnode "FPGA I/O Method Node"("FPGA I/O In"=refnum<k21> "Connector0/DIO8" ("APD 2 DO"), "Timeout"=-1) -> ()  [unwired: 2 out]
          }
          frame #1 {
            n113 = local read "APD2 int gate"() -> (w228:bool)
            n114 = case shown="True" w228 {
              frame False {
              }
              frame True {
                n115 = local read "APD2 out state"() -> (w229:bool)
                n116 = case shown="False" w229 {
                  frame False {
                    n117 = local read "APD 2 Counts 0"() -> (w231:u32)
                    n118 = Increment(x=w231) -> (x+1=→"APD 2 Counts 0":u32)
                  }
                  frame True {
                    n119 = local read "APD 2 Counts 1"() -> (w233:u32)
                    n120 = Increment(x=w233) -> (x+1=→"APD 2 Counts 1":u32)
                  }
                }
              }
            }
          }
        }
      }
      n121 = while "APD 1 Counter" {
        tunnel: w215 -> [_]
        stop <- FALSE stop-if-true
        n122 = flat-sequence {
          frame #0 {
            n123 = xnode "FPGA I/O Method Node"("FPGA I/O In"=refnum<k21> "Connector0/DIO4" ("APD 1 DO"), "Timeout"=-1) -> ()  [unwired: 2 out]
          }
          frame #1 {
            n124 = local read "APD1 int gate"() -> (w219:bool)
            n125 = case shown="True" w219 {
              frame False {
              }
              frame True {
                n126 = local read "APD1 out state"() -> (w220:bool)
                n127 = case shown="True" w220 {
                  frame False {
                    n128 = local read "APD 1 Counts 0"() -> (w222:u32)
                    n129 = Increment(x=w222) -> (x+1=→"APD 1 Counts 0":u32)
                  }
                  frame True {
                    n130 = local read "APD 1 Counts 1"() -> (w224:u32)
                    n131 = Increment(x=w224) -> (x+1=→"APD 1 Counts 1":u32)
                  }
                }
              }
            }
          }
        }
      }
    }
    frame Enabled {
    }
  }
  n132 = disable-structure shown="Disabled" {
    disable-tunnel: w4 -> [w234 _]
    frame Disabled {
      w235 = u16 0
      n133 = while "Green and red fluorescent laser interlacing (Current AO to IA 532 nm AOM ME amp)." {
        shift-right: [w315] -> _
        shift-left: w234 -> [w318]
        shift-right: [w312] -> _
        shift-left: w235 -> [w310]
        shift-right: [w309] -> _
        shift-left: w235 -> [w308]
        stop <- FALSE stop-if-true
        n134 = flat-sequence {
          tunnel: w318 -> [w322]
          tunnel: [w323] -> w317
          tunnel: [w322] -> w316
          tunnel: [w321] -> w311
          tunnel: w310 -> [w321]
          tunnel: w308 -> [w320]
          tunnel: [w320] -> w307
          tunnel: [w327] -> w314
          tunnel: w317 -> [w327]
          tunnel: [w326] -> w313
          tunnel: w316 -> [w326]
          tunnel: w311 -> [w325]
          tunnel: w307 -> [w324]
          tunnel: [w355] -> w315
          tunnel: [w371] -> w312
          tunnel: w314 -> [w382]
          tunnel: w313 -> [w379]
          tunnel: [w340] -> w309
          frame #0 {
            n135 = call "Loop Timer10"("Count(Ticks)"=w322) -> ("Tick Count(Ticks)"=w323:u16)
          }
          frame #1 {
            n136 = xnode "FPGA I/O Node"("Chassis2/Mod4/AO0"=w325, "Chassis2/Mod4/AO1"=w324) -> ()  [unwired: 2 in, 2 out]
          }
          frame #2 {
            # "IF RF synth BD does green, never run FB"
            # "ALEX variable is used by APD acquisition loop\nto turn lasers ON/OFF."
            # "Design note:\n\nThese two laser controls are in the same loop\nbecause the expansion current AI cannot separately\ntime the outputs fast enough for us.  Apparently\nit is because of communication time between the\nexpansion card and the fpga.\n\nSo the two analog control signals have the same timing\nand profile, but independent amplitudes to independently\ncontrol the intensity and feedback for each laser."
            n137 = feedback #12(TRUE) -> (w337:bool)
            n138 = Not(x=w337) -> (.not. x?=w338:bool)
            n139 = feedback-in #12(w338) -> ()
            n140 = Subtract(x="Green interlace OFF count 2", y="Green int current ON count adj") -> (x-y=w364:u16)
            n141 = feedback-in #13(w382) -> ()
            n142 = feedback #13(w382) -> (w381:u16)
            n143 = Add(x="Green int current ON count adj", y="Green interlace ON count 2") -> (x+y=w365:u16)
            n144 = Subtract(x=w382, y=w381) -> (x-y=w380:u16)
            n145 = Select(t=w365, s=w338, f=w364) -> (s? t:f=w376:u16)
            n146 = Subtract(x=w380, y=w379) -> (x-y=w348:u16)
            n147 = case shown="2" "RI Operating Mode 2" {
              tunnel: [TRUE FALSE w388] -> w333
              tunnel: w337 -> [_ _ w385]
              frame 0, Default {
              }
              frame 1 {
              }
              frame 2 {
                n148 = Not(x=w385) -> (.not. x?=w387:bool)
                n149 = Select(t=w387, s="Invert RI 2", f=w385) -> (s? t:f=w388:bool)
              }
            }
            n150 = Subtract(x=w376, y=w348) -> (x-y=w359:u16)
            n151 = case shown="2" "Operating Mode 2" {
              tunnel: [TRUE FALSE w422] -> w335
              tunnel: w337 -> [_ _ w419]
              frame 0, Default {
              }
              frame 1 {
              }
              frame 2 {
                n152 = Not(x=w419) -> (.not. x?=w421:bool)
                n153 = Select(t=w421, s="Invert GI 2", f=w419) -> (s? t:f=w422:bool)
              }
            }
            n154 = Number To Boolean Array(number=w348) -> (Boolean array=w349:bool[])
            n155 = Boolean To (0,1)(Boolean="+ phase (GI) 2") -> (0, 1=w361:i16)
            n156 = Or Array Elements(Boolean array=w349) -> (logical OR=w347:bool)
            n157 = local read item#-1() -> (w332)
            n158 = Boolean To (0,1)(Boolean=w347) -> (0, 1=w354:i16)
            n159 = Multiply(x=w361, y="Phase count adjustment (GI) 2") -> (x*y=w357:i16)
            n160 = local read item#-1() -> (w334)
            n161 = local read "RF synth bd controls green"() -> (w329:bool)
            n162 = To Unsigned Byte Integer(number=w354) -> (unsigned 8bit integer=w350:u8)
            n163 = And(x=w332, y=w333) -> (x .and. y?=w331:bool)
            n164 = Add(x=w359, y=w357) -> (x+y=w355:u16)
            n165 = feedback #14(u8 0) -> (w352:u8)
            n166 = Add(x=w350, y=w352) -> (x+y=w351:u8)
            "GI Late Counter 2" <- w351
            n167 = feedback-in #14(w351) -> ()
            n168 = feedback #15(i16 0) -> (w358:i16)
            n169 = Subtract(x=w358, y=w357) -> (x-y=w356:i16)
            "GI Relative phase 2" <- w356
            n170 = feedback-in #15(w356) -> ()
            n171 = And(x=w335, y=w334) -> (x .and. y?=w336:bool)
            n172 = And(x=w336, y="Green FB On/Off") -> (x .and. y?=w366:bool)
            "green FB running" <- w366
            n173 = And(x=w331, y="Red FB On/Off") -> (x .and. y?=w346:bool)
            n174 = Not(x=w329) -> (.not. x?=w328:bool)
            n175 = case shown="True" w346 {
              tunnel: "RI Current Out" -> [w389 _]
              tunnel: [w389 w398] -> w342
              frame False {
              }
              frame True {
                n176 = local read "Red FB Intensity"() -> (w394:i16)
                n177 = Bundle("P4"="P4", "I4"="I4", "D4"="D4") -> (w390:cluster{"P4":i16, "I4":i16, "D4":i16})  [unwired: 1 in]
                n178 = call "Slower PID.vi"("process variable"=w394, "reset?"="Red FB Reset", "setpoint"="Red FB Setpoint", "PID gains (x 2^8)"=w390, "output range"=cluster{"output high":i16, "output low":i16} {"output high"=32767, "output low"=-32768} ("Green FB output range")) -> ("output"=w401:i16)  [unwired: 10 out]
                n179 = To Long Integer(number=w401) -> (32bit integer=w395:i32)
                n180 = Add(x=w395, y=32768) -> (x+y=w397:i32)
                n181 = To Unsigned Word Integer(number=w397) -> (unsigned 16bit integer=w398:u16)
              }
            }
            n182 = And(x=w366, y=w328) -> (x .and. y?=w330:bool)
            n183 = case shown="True" w330 {
              tunnel: "Current Out" -> [w403 w404]
              tunnel: [w403 w404] -> w370
              frame False {
              }
              frame True {
                n184 = disable-structure shown="Disabled" {
                  frame Disabled {
                    n185 = local read "Green FB Sum"() -> (w409:i16)
                    n186 = Bundle("P3"="P3", "I3"="I3", "D3"="D3") -> (w405:cluster{"P3":i16, "I3":i16, "D3":i16})  [unwired: 1 in]
                    n187 = call "Slower PID.vi"("process variable"=w409, "reset?"="Green FB Reset", "setpoint"="Green FB Setpoint", "PID gains (x 2^8)"=w405, "output range"=cluster{"output high":i16, "output low":i16} {"output high"=32767, "output low"=-32768} ("Green FB output range")) -> ("output"=w415:i16)  [unwired: 10 out]
                    n188 = To Long Integer(number=w415) -> (32bit integer=w410:i32)
                    n189 = Add(x=w410, y=32768) -> (x+y=w412:i32)
                    n190 = To Unsigned Word Integer(number=w412) -> ()  [unwired: 1 out]
                  }
                  frame Enabled {
                  }
                }
              }
            }
            n191 = Boolean To (0,1)(Boolean=w331) -> (0, 1=w341:i16)
            n192 = To Unsigned Word Integer(number=w341) -> (unsigned 16bit integer=w343:u16)
            n193 = Boolean To (0,1)(Boolean=w336) -> (0, 1=w372:i16)
            n194 = To Unsigned Word Integer(number=w372) -> (unsigned 16bit integer=w369:u16)
            n195 = Compound Arithmetic op=MULTIPLY(w343, w342) -> (w340:u16)
            n196 = Compound Arithmetic op=MULTIPLY(w369, w370) -> (w371:u16)
          }
        }
      }
      n197 = while "Blue fluorescent laser interlacing (AO control direct to laser)." {
        shift-right: [w242] -> _
        shift-left: w234 -> [w245]
        shift-right: [w239] -> _
        shift-left: i16 0 -> [w237]
        stop <- FALSE stop-if-true
        n198 = flat-sequence {
          tunnel: w245 -> [w248]
          tunnel: [w249] -> w244
          tunnel: [w248] -> w243
          tunnel: [w247] -> w238
          tunnel: w237 -> [w247]
          tunnel: [w252] -> w241
          tunnel: w244 -> [w252]
          tunnel: [w251] -> w240
          tunnel: w243 -> [w251]
          tunnel: w238 -> [w250]
          tunnel: [w262] -> w242
          tunnel: [w278] -> w239
          tunnel: w241 -> [w290]
          tunnel: w240 -> [w287]
          frame #0 {
            n199 = call "Loop Timer13"("Count(Ticks)"=w248) -> ("Tick Count(Ticks)"=w249:u16)
          }
          frame #1 {
            n200 = xnode "FPGA I/O Node"("Connector0/AO3"=w250) -> ()  [unwired: 1 in, 1 out]
          }
          frame #2 {
            n201 = Subtract(x="Blue OFF count (AO)", y="Blue current ON count adj (AO)") -> (x-y=w271:u16)
            n202 = feedback-in #16(w290) -> ()
            n203 = feedback #16(w290) -> (w289:u16)
            n204 = Add(x="Blue current ON count adj (AO)", y="Blue ON count (AO)") -> (x+y=w272:u16)
            n205 = Subtract(x=w290, y=w289) -> (x-y=w288:u16)
            n206 = Subtract(x=w288, y=w287) -> (x-y=w255:u16)
            n207 = Number To Boolean Array(number=w255) -> (Boolean array=w256:bool[])
            n208 = Boolean To (0,1)(Boolean="+ phase (BI AO)") -> (0, 1=w268:i16)
            n209 = Or Array Elements(Boolean array=w256) -> (logical OR=w254:bool)
            n210 = Boolean To (0,1)(Boolean=w254) -> (0, 1=w261:i16)
            n211 = Multiply(x=w268, y="Phase count adjustment (BI AO)") -> (x*y=w264:i16)
            n212 = To Unsigned Byte Integer(number=w261) -> (unsigned 8bit integer=w257:u8)
            n213 = feedback #17(u8 0) -> (w259:u8)
            n214 = Add(x=w257, y=w259) -> (x+y=w258:u8)
            "BI Late Counter (AO)" <- w258
            n215 = feedback-in #17(w258) -> ()
            n216 = feedback #18(i16 0) -> (w265:i16)
            n217 = Subtract(x=w265, y=w264) -> (x-y=w263:i16)
            "BI Relative phase (AO)" <- w263
            n218 = feedback-in #18(w263) -> ()
            n219 = feedback #19(TRUE) -> (w282:bool)
            n220 = case shown="2" "BI Operating Mode (AO)" {
              tunnel: [TRUE FALSE w306] -> w273
              tunnel: w282 -> [_ _ w303]
              frame 0, Default {
              }
              frame 1 {
              }
              frame 2 {
                n221 = Not(x=w303) -> (.not. x?=w305:bool)
                n222 = Select(t=w305, s="Invert BI (AO)", f=w303) -> (s? t:f=w306:bool)
              }
            }
            n223 = And(x=w273, y="Blue FB On/Off") -> (x .and. y?=w274:bool)
            n224 = case shown="True" w274 {
              tunnel: "BI Current Out" -> [w291 _]
              tunnel: [w291 w293] -> w277
              frame False {
              }
              frame True {
                n225 = local read "Blue Intensity"() -> (w292:i16)
                n226 = Bundle("P5"="P5", "I5"="I5", "D5"="D5") -> (w294:cluster{"P5":i16, "I5":i16, "D5":i16})  [unwired: 1 in]
                n227 = call "Slower PID.vi"("process variable"=w292, "reset?"="Blue FB Reset", "setpoint"="Blue FB Setpoint", "PID gains (x 2^8)"=w294, "output range"=cluster{"output high":i16, "output low":i16} {"output high"=32767, "output low"=0} ("Green FB output range")) -> ("output"=w293:i16)  [unwired: 10 out]
              }
            }
            n228 = Not(x=w282) -> (.not. x?=w279:bool)
            n229 = Select(t=w272, s=w279, f=w271) -> (s? t:f=w284:u16)
            n230 = Subtract(x=w284, y=w255) -> (x-y=w266:u16)
            n231 = Add(x=w266, y=w264) -> (x+y=w262:u16)
            n232 = feedback-in #19(w279) -> ()
            n233 = Boolean To (0,1)(Boolean=w273) -> (0, 1=w253:i16)
            n234 = Multiply(x=w253, y=w277) -> (x*y=w278:i16)
          }
        }
      }
    }
    frame Enabled {
    }
  }
  n235 = while "fluorescent laser interlacing (DO)." {
    shift-right: [w429] -> _
    shift-left: w4 -> [w434]
    shift-right: [w428] -> _
    shift-left: w15 -> [w426]
    shift-right: [w425] -> _
    shift-left: u8 0 -> [w423]
    stop <- FALSE stop-if-true
    n236 = flat-sequence {
      tunnel: w434 -> [w438]
      tunnel: [w439] -> w432
      tunnel: [w438] -> w430
      tunnel: [w437] -> w427
      tunnel: w426 -> [w437]
      tunnel: [w436] -> w424
      tunnel: w423 -> [w436]
      tunnel: [w443] -> w433
      tunnel: w432 -> [w443]
      tunnel: [w442] -> w431
      tunnel: w430 -> [w442]
      tunnel: w427 -> [w441]
      tunnel: w424 -> [w440]
      tunnel: [w472] -> w429
      tunnel: w433 -> [w491]
      tunnel: w431 -> [w488]
      tunnel: [w481] -> w428
      tunnel: [w453] -> w425
      frame #0 {
        n237 = call "Loop Timer4"("Count(Ticks)"=w438) -> ("Tick Count(Ticks)"=w439:u16)
      }
      frame #1 {
        n238 = case shown="2" w440 {
          tunnel: w441 -> [w445 w447 w449]
          frame 0, Default {
            w444 = FALSE
            n239 = xnode "FPGA I/O Node"("Connector0/DIO9"=w445, "Connector0/DIO11"=w444, "Connector0/DIO13"=w444) -> ()  [unwired: 3 in, 3 out]
          }
          frame 1 {
            w446 = FALSE
            n240 = xnode "FPGA I/O Node"("Connector0/DIO9"=w446, "Connector0/DIO11"=w447, "Connector0/DIO13"=w446) -> ()  [unwired: 3 in, 3 out]
          }
          frame 2 {
            w448 = FALSE
            n241 = xnode "FPGA I/O Node"("Connector0/DIO9"=w448, "Connector0/DIO11"=w448, "Connector0/DIO13"=w449) -> ()  [unwired: 3 in, 3 out]
          }
        }
      }
      frame #2 {
        # "Laser counting"
        n242 = feedback-in #20(w491) -> ()
        n243 = feedback #20(w491) -> (w490:u16)
        n244 = Subtract(x=w491, y=w490) -> (x-y=w489:u16)
        n245 = Subtract(x=w489, y=w488) -> (x-y=w465:u16)
        n246 = Number To Boolean Array(number=w465) -> (Boolean array=w466:bool[])
        n247 = Or Array Elements(Boolean array=w466) -> (logical OR=w464:bool)
        n248 = feedback #21(u8 0) -> (w462:u8)
        n249 = Increment(x=w462) -> (x+1=w459:u8)
        n250 = Less?(x=u8 5, y=w459) -> (x < y?=w460:bool)
        n251 = Select(t=u8 0, s=w460, f=w459) -> (s? t:f=w451:u8)
        n252 = feedback-in #21(w451) -> ()
        n253 = Boolean To (0,1)(Boolean=w464) -> (0, 1=w471:i16)
        n254 = Quotient & Remainder(x=w451, y=u8 2) -> (floor(x/y)=w450:u8)  [unwired: 1 out]
        n255 = To Unsigned Byte Integer(number=w471) -> (unsigned 8bit integer=w468:u8)
        n256 = feedback #22(u8 0) -> (w469:u8)
        n257 = Add(x=w468, y=w469) -> (x+y=w467:u8)
        "GI Late Counter" <- w467
        n258 = feedback-in #22(w467) -> ()
        n259 = Boolean To (0,1)(Boolean="+ phase (GI)") -> (0, 1=w477:i16)
        n260 = Multiply(x=w477, y="Phase count adjustment (GI)") -> (x*y=w474:i16)
        n261 = feedback #23(i16 0) -> (w475:i16)
        n262 = Subtract(x=w475, y=w474) -> (x-y=w473:i16)
        "GI Relative phase" <- w473
        n263 = feedback-in #23(w473) -> ()
        n264 = feedback #24(TRUE) -> (w484:bool)
        n265 = case shown="2" "Operating Mode" {
          tunnel: [TRUE FALSE w581] -> w481
          tunnel: w484 -> [_ _ w578]
          frame 0, Default {
          }
          frame 1 {
          }
          frame 2 {
            n266 = Not(x=w578) -> (.not. x?=w580:bool)
            n267 = Select(t=w580, s="Invert GI", f=w578) -> (s? t:f=w581:bool)
          }
        }
        n268 = Not(x=w484) -> (.not. x?=w480:bool)
        n269 = case shown="2" w450 {
          tunnel: "FL interlace ON count 0" -> [w501 w528 w555]
          tunnel: "FL interlace OFF count 0" -> [w500 w527 w554]
          tunnel: w480 -> [w499 w526 w557]
          tunnel: [w497 w525 w553] -> w478
          tunnel: w465 -> [w498 w529 w556]
          tunnel: "Fl interlace ON count 1" -> [w496 w524 w552]
          tunnel: "FL interlace OFF count 1" -> [w495 w523 w551]
          tunnel: "FL interlace ON count 2" -> [w494 w522 w550]
          tunnel: "FL interlace OFF count 2" -> [w493 w521 w549]
          tunnel: ["Laser choice 0" "Laser choice 1" "Laser choice 2"] -> w453
          frame 0, Default {
            n270 = case shown="1" "Laser choice 0" {
              tunnel: w501 -> [w506 _ _]
              tunnel: w500 -> [w505 _ _]
              tunnel: w499 -> [w504 w510 w516]
              tunnel: w498 -> [w503 w509 w515]
              tunnel: [w502 w508 w514] -> w497
              tunnel: w496 -> [_ w512 _]
              tunnel: w495 -> [_ w511 _]
              tunnel: w494 -> [_ _ w518]
              tunnel: w493 -> [_ _ w517]
              frame 0, Default {
                n271 = Select(t=w506, s=w504, f=w505) -> (s? t:f=w507:u16)
                n272 = Subtract(x=w507, y=w503) -> (x-y=w502:u16)
              }
              frame 1 {
                n273 = Select(t=w512, s=w510, f=w511) -> (s? t:f=w513:u16)
                n274 = Subtract(x=w513, y=w509) -> (x-y=w508:u16)
              }
              frame 2 {
                n275 = Select(t=w518, s=w516, f=w517) -> (s? t:f=w519:u16)
                n276 = Subtract(x=w519, y=w515) -> (x-y=w514:u16)
              }
            }
          }
          frame 1 {
            n277 = case shown="2" "Laser choice 1" {
              tunnel: w528 -> [w534 _ _]
              tunnel: w527 -> [w533 _ _]
              tunnel: w526 -> [w532 w538 w544]
              tunnel: w529 -> [w531 w537 w543]
              tunnel: [w530 w536 w542] -> w525
              tunnel: w524 -> [_ w540 _]
              tunnel: w523 -> [_ w539 _]
              tunnel: w522 -> [_ _ w546]
              tunnel: w521 -> [_ _ w545]
              frame 0, Default {
                n278 = Select(t=w534, s=w532, f=w533) -> (s? t:f=w535:u16)
                n279 = Subtract(x=w535, y=w531) -> (x-y=w530:u16)
              }
              frame 1 {
                n280 = Select(t=w540, s=w538, f=w539) -> (s? t:f=w541:u16)
                n281 = Subtract(x=w541, y=w537) -> (x-y=w536:u16)
              }
              frame 2 {
                n282 = Select(t=w546, s=w544, f=w545) -> (s? t:f=w547:u16)
                n283 = Subtract(x=w547, y=w543) -> (x-y=w542:u16)
              }
            }
          }
          frame 2 {
            n284 = case shown="2" "Laser choice 2" {
              tunnel: w555 -> [w562 _ _]
              tunnel: w554 -> [w561 _ _]
              tunnel: w557 -> [w560 w566 w572]
              tunnel: w556 -> [w559 w565 w571]
              tunnel: [w558 w564 w570] -> w553
              tunnel: w552 -> [_ w568 _]
              tunnel: w551 -> [_ w567 _]
              tunnel: w550 -> [_ _ w574]
              tunnel: w549 -> [_ _ w573]
              frame 0, Default {
                n285 = Select(t=w562, s=w560, f=w561) -> (s? t:f=w563:u16)
                n286 = Subtract(x=w563, y=w559) -> (x-y=w558:u16)
              }
              frame 1 {
                n287 = Select(t=w568, s=w566, f=w567) -> (s? t:f=w569:u16)
                n288 = Subtract(x=w569, y=w565) -> (x-y=w564:u16)
              }
              frame 2 {
                n289 = Select(t=w574, s=w572, f=w573) -> (s? t:f=w575:u16)
                n290 = Subtract(x=w575, y=w571) -> (x-y=w570:u16)
              }
            }
          }
        }
        n291 = Add(x=w478, y=w474) -> (x+y=w472:u16)
        n292 = feedback-in #24(w480) -> ()
      }
    }
  }
  n293 = while "DAQ AI set 1" {
    shift-right: [w582] -> _
    shift-left: w4 -> [w587]
    stop <- FALSE stop-if-true
    n294 = flat-sequence {
      tunnel: w587 -> [w597]
      tunnel: [w598] -> w585
      tunnel: [w597] -> w584
      tunnel: [w608] -> w595
      tunnel: [w607] -> w594
      tunnel: [w606] -> w593
      tunnel: [w605] -> w592
      tunnel: [w604] -> w591
      tunnel: [w603] -> w590
      tunnel: [w602] -> w589
      tunnel: [w601] -> w588
      tunnel: [w600] -> w586
      tunnel: w585 -> [w600]
      tunnel: w584 -> [w599]
      tunnel: [w599] -> w583
      tunnel: [w640] -> w582
      tunnel: w595 -> [w666]
      tunnel: w594 -> [w632]
      tunnel: w593 -> [w633]
      tunnel: w592 -> [w610]
      tunnel: w591 -> [w656]
      tunnel: w590 -> [w655]
      tunnel: w589 -> [w654]
      tunnel: w588 -> [w653]
      tunnel: w586 -> [w650]
      tunnel: w583 -> [w647]
      frame #0 {
        n295 = call "Loop Timer3"("Count(Ticks)"=w597) -> ("Tick Count(Ticks)"=w598:u16)
      }
      frame #1 {
        # "Signal changed to DIO15 to ease\nmeasurement in the room - change\nback for large code"
        n296 = xnode "FPGA I/O Node"("Connector0/DIO15"=TRUE ("Connector1/DIO33")) -> ("Connector0/AI0"=w608:i16, "Connector0/AI1"=w607:i16, "Connector0/AI2"=w606:i16, "Connector0/AI3"=w605:i16, "Connector0/AI4"=w604:i16, "Connector0/AI5"=w603:i16, "Connector0/AI6"=w602:i16, "Connector0/AI7"=w601:i16)  [unwired: 9 in, 9 out]
      }
      frame #2 {
        w636 = FALSE ("AI to FIFO")
        # "Normalize by trap bead QPD sum, AI3"
        # "Adjust phase after data acquired if button pressed"
        n297 = feedback #25(i16 1) -> (w659:i16)
        n298 = Increment(x=w659) -> (x+1=w665:i16)
        n299 = Scale By Power Of 2(n="AI1 X Scale", x=w632) -> (x*2^n=w630:i16)
        n300 = Greater?(x=w665, y="N of AI1 Int Acq Sets") -> (0:w662:bool)
        n301 = Select(t=i16 1, s=w662, f=w665) -> (s? t:f=w664:i16)
        n302 = feedback-in #25(w664) -> ()
        n303 = Divide(x=w630, y=w610) -> (x/y=w629:fxp<+/-,16,1>)
        n304 = feedback #26(w636) -> (w634:bool)
        n305 = feedback #27(w636) -> (w652:bool)
        n306 = case shown="1, Default" w659 {
          tunnel: w633 -> [w691 w698 _]
          tunnel: ["Set 1" "Set 2" "Set 3"] -> w657
          tunnel: ["AI to FIFO" w700 w705] -> w651
          tunnel: w652 -> [_ w700 w705]
          tunnel: ["Trap Pos to FIFO" w699 w704] -> w635
          tunnel: w634 -> [_ w699 w704]
          tunnel: w629 -> [w690 w697 _]
          tunnel: [w689 w695 FALSE] -> w616
          tunnel: [w688 w696 u64 0 ("BD1 Frequency Out 2")] -> w615
          frame 1, Default {
            n307 = local read "BD1 Frequency Out 1"() -> (w688:u64)
            n308 = Compound Arithmetic op=AND("Trap Pos to FIFO", "Set 1", "AI to FIFO") -> (w689:bool)
            "AI2 Y Sum Set 1" <- w691
            "AI1 X Set 1" <- w690
          }
          frame 2 {
            n309 = local read "BD1 Frequency Out 2"() -> (w696:u64)
            n310 = Compound Arithmetic op=AND(w699, "Set 2", w700) -> (w695:bool)
            "AI2 Y Sum Set 2" <- w698
            "AI1 X Set 2" <- w697
          }
          frame 3 {
          }
        }
        n311 = And(x=w657, y=w651) -> (x .and. y?=w658:bool)
        n312 = case shown="True" w658 {
          tunnel: w666 -> [_ w719]
          tunnel: w632 -> [_ w718]
          tunnel: w633 -> [_ w717]
          tunnel: w610 -> [_ w716]
          tunnel: w656 -> [_ w715]
          tunnel: w655 -> [_ w714]
          tunnel: w654 -> [_ w713]
          tunnel: w653 -> [_ w712]
          tunnel: 0 ("DMA buffer timeout") -> [_ w721]
          frame False {
          }
          frame True {
            n313 = Build Array(w719, w718, w717, w716, w715, w714, w713, w712) -> (w720:i16[])
            n314 = for {
              tunnel: w720 -> [w723] mode=indexing
              tunnel: w721 -> [w724]
              tunnel: [w722] -> w710 mode=indexing
              n315 = xnode ("FIFO Write")("Element"=w723, "Timeout"=w724) -> ("Timed Out?"=w722:bool)  [unwired: 1 in, 1 out]
            }
            n316 = Or Array Elements(Boolean array=w710) -> (logical OR=w707:bool)
            n317 = Boolean To (0,1)(Boolean=w707) -> (0, 1=w709:i16)
            n318 = feedback #28(u16 0) -> (w708:u16)
            n319 = Add(x=w709, y=w708) -> (x+y=w706:u16)
            "Trap AI FIFO Timeout" <- w706
            n320 = feedback-in #28(w706) -> ()
          }
        }
        n321 = feedback-in #26(w635) -> ()
        n322 = feedback-in #27(w651) -> ()
        n323 = local read "Piezo X out"() -> (w612:i16)
        n324 = local read "Piezo Y out"() -> (w611:i16)
        n325 = case shown="True" w616 {
          tunnel: w615 -> [_ w674]
          tunnel: [u8 0 w671] -> w614
          tunnel: w612 -> [_ w670]
          tunnel: w611 -> [_ w669]
          frame False {
          }
          frame True {
            n326 = Split Number(x=w674) -> (hi(x)=w675:u32, lo(x)=w676:u32)
            n327 = Split Number(x=w675) -> (lo(x)=w677:u16)  [unwired: 1 out]
            n328 = Split Number(x=w676) -> (hi(x)=w678:u16, lo(x)=w679:u16)
            n329 = Build Array "BD 1 nu Stack"(w677, w678, w679, w670, w669) -> (w673:u16[])
            n330 = for {
              tunnel: w673 -> [w686] mode=indexing
              shift-right: [w682] -> w671
              shift-left: u8 0 -> [w683]
              n331 = xnode ("FIFO Method Node")("Element"=w686, "Timeout"="Trap FIFO Set Timeout") -> ("Timed Out?"=w685:bool)  [unwired: 1 in, 1 out]
              n332 = Boolean To (0,1)(Boolean=w685) -> (0, 1=w684:i16)
              n333 = To Unsigned Byte Integer(number=w684) -> (unsigned 8bit integer=w681:u8)
              n334 = Add(x=w681, y=w683) -> (x+y=w682:u8)
            }
          }
        }
        n335 = To Unsigned Word Integer(number=w614) -> (unsigned 16bit integer=w613:u16)
        n336 = feedback #29(u16 0) -> (w627:u16)
        n337 = Add(x=w613, y=w627) -> (x+y=w626:u16)
        "Trap Pos FIFO Timeout" <- w626
        n338 = feedback-in #29(w626) -> ()
        n339 = feedback-in #30(w650) -> ()
        n340 = feedback #30(w650) -> (w649:u16)
        n341 = Subtract(x=w650, y=w649) -> (x-y=w648:u16)
        n342 = xnode "FPGA I/O Node"("Connector0/DIO15"=FALSE ("Connector1/DIO34")) -> ()  [unwired: 1 in, 1 out]
        n343 = Subtract(x=w648, y=w647) -> (x-y=w618:u16)
        n344 = Boolean To (0,1)(Boolean="+ phase") -> (0, 1=w643:i16)
        n345 = Multiply(x=w643, y="Phase count adjustment") -> (x*y=w637:i16)
        n346 = Subtract(x="ai count", y=w618) -> (x-y=w641:u16)
        n347 = Number To Boolean Array(number=w618) -> (Boolean array=w619:bool[])
        n348 = feedback #31(i16 0) -> (w639:i16)
        n349 = Add(x=w641, y=w637) -> (x+y=w640:u16)
        n350 = Subtract(x=w639, y=w637) -> (x-y=w638:i16)
        "Relative phase" <- w638
        n351 = feedback-in #31(w638) -> ()
        n352 = Or Array Elements(Boolean array=w619) -> (logical OR=w617:bool)
        n353 = Boolean To (0,1)(Boolean=w617) -> (0, 1=w624:i16)
        n354 = To Unsigned Byte Integer(number=w624) -> (unsigned 8bit integer=w621:u8)
        n355 = feedback #32(u8 0) -> (w622:u8)
        n356 = Add(x=w621, y=w622) -> (x+y=w620:u8)
        "AI Late Counter" <- w620
        n357 = feedback-in #32(w620) -> ()
      }
    }
  }
  n358 = while "MCL stage control" {
    shift-right: [w748] -> _
    shift-left: w4 -> [w751]
    shift-right: [w741] -> _
    shift-left: w13 -> [w738]
    shift-right: [w740] -> _
    shift-left: w12 -> [w736]
    shift-right: [w735] -> _
    shift-left: w11 -> [w730]
    shift-right: [w733] -> _
    shift-left: w11 -> [w725]
    shift-right: [w731] -> _
    shift-left: w11 -> [w727]
    stop <- FALSE stop-if-true
    n359 = flat-sequence {
      tunnel: w751 -> [w758]
      tunnel: [w759] -> w747
      tunnel: [w758] -> w745
      tunnel: [w757] -> w739
      tunnel: w738 -> [w757]
      tunnel: [w756] -> w737
      tunnel: w736 -> [w756]
      tunnel: w730 -> [w755]
      tunnel: [w755] -> w729
      tunnel: [w754] -> w728
      tunnel: w727 -> [w754]
      tunnel: [w753] -> w726
      tunnel: w725 -> [w753]
      tunnel: w747 -> [w766]
      tunnel: [w766] -> w746
      tunnel: w745 -> [w765]
      tunnel: [w765] -> w744
      tunnel: w739 -> [w764]
      tunnel: w737 -> [w763]
      tunnel: w729 -> [w762]
      tunnel: w728 -> [w761]
      tunnel: w726 -> [w760]
      tunnel: w746 -> [w780]
      tunnel: w744 -> [w779]
      tunnel: [w780] -> w750
      tunnel: [w779] -> w749
      tunnel: [w778] -> w743
      tunnel: [w777] -> w742
      tunnel: [w769] -> w734
      tunnel: [w767] -> w732
      tunnel: [w887] -> w748
      tunnel: w750 -> [w894]
      tunnel: w749 -> [w891]
      tunnel: w743 -> [w889]
      tunnel: w742 -> [w888]
      tunnel: [w889] -> w741
      tunnel: [w888] -> w740
      tunnel: [w870] -> w735
      tunnel: w734 -> [w870]
      tunnel: [w869] -> w733
      tunnel: w732 -> [w869]
      tunnel: ["Piezo Trap ON/Off (AO3)"] -> w731
      frame #0 {
        n360 = call "Loop Timer5"("Count(Ticks)"=w758) -> ("Tick Count(Ticks)"=w759:u32)
      }
      frame #1 {
        n361 = xnode "FPGA I/O Node"("Connector0/AO1"=w764, "Connector0/AO2"=w763, "Connector0/AO3"=w761, "Connector0/AO4"=w762, "Connector0/AO5"=w760) -> ()  [unwired: 5 in, 5 out]
      }
      frame #2 {
        n362 = local read "Scanning MCL"() -> (w792:bool)
        n363 = Or(x=w792, y="Start scan (MCL)") -> (x .or. y?=w787:bool)
        n364 = Not(x="Abort scan (MCL)") -> (.not. x?=w785:bool)
        n365 = And(x=w785, y=w787) -> (x .and. y?=w784:bool)
        n366 = case "Raster scan" shown="False" w784 {
          tunnel: [w825 w868] -> w789
          tunnel: "Start scan (MCL)" -> [_ w853]
          tunnel: [w825 w829] -> w773
          frame False {
            w825 = i16 0
            n367 = local write "Scanning MCL"(FALSE ("scanning")) -> ()
          }
          frame True {
            w839 = i16 0
            w838 = u64 0
            # "scan incr."
            # "freq. incr. mult."
            # "count steps"
            # "count number of cycles"
            n368 = feedback #33(w838) -> (w865:u64)
            n369 = Select(t=w838, s=w853, f=w865) -> (s? t:f=w867:u64)
            n370 = Increment(x=w867) -> (x+1=w864:u64)
            n371 = Greater?(x="Cycles per step (MCL)", y=w864) -> (0:w848:bool)
            n372 = Select(t=w864, s=w848, f=w838) -> (s? t:f=w863:u64)
            n373 = feedback-in #33(w863) -> ()
            n374 = feedback #34(w838) -> (w862:u64)
            n375 = Select(t=w838, s=w853, f=w862) -> (s? t:f=w857:u64)
            n376 = Increment(x=w857) -> (x+1=w861:u64)
            n377 = Add(x="Scan steps (MCL)", y="Scan steps (MCL)") -> (x+y=w860:u64)
            n378 = Select(t=w857, s=w848, f=w861) -> (s? t:f=w843:u64)
            n379 = Greater?(x=w860, y=w843) -> (0:w842:bool)
            n380 = Select(t=w843, s=w842, f=w838) -> (s? t:f=w858:u64)
            n381 = feedback-in #34(w858) -> ()
            n382 = Equal?(x="Scan steps (MCL)", y=w843) -> (x = y?=w847:bool)
            n383 = Greater?(x="Scan steps (MCL)", y=w857) -> (0:w856:bool)
            n384 = feedback #35(w839) -> (w859:i16)
            n385 = Select(t=w839, s=w853, f=w859) -> (s? t:f=w845:i16)
            n386 = Increment(x=w845) -> (x+1=w855:i16)
            n387 = Decrement(x=w845) -> (x-1=w854:i16)
            n388 = Select(t=w855, s=w856, f=w854) -> (s? t:f=w846:i16)
            n389 = Select(t=w845, s=w847, f=w846) -> (s? t:f=w844:i16)
            n390 = Select(t=w845, s=w848, f=w844) -> (s? t:f=w840:i16)
            n391 = Select(t=w840, s=w842, f=w839) -> (s? t:f=w841:i16)
            n392 = feedback-in #35(w841) -> ()
            n393 = feedback #36(w838) -> (w852:u64)
            n394 = Select(t=w838, s=w853, f=w852) -> (s? t:f=w827:u64)
            n395 = Increment(x=w827) -> (x+1=w849:u64)
            n396 = Select(t=w827, s=w842, f=w849) -> (s? t:f=w828:u64)
            n397 = Greater?(x="Number of scans (MCL)", y=w828) -> (0:w835:bool)
            n398 = Multiply(x="Scan freq.  increment (MCL)", y=w845) -> (x*y=w868:i16)
            n399 = Select(t=TRUE, s="Cont. Scan (MCL)", f=w835) -> (s? t:f=w834:bool)
            "Scanning MCL" <- w834
            n400 = Select(t=w828, s=w834, f=w838) -> (s? t:f=w850:u64)
            n401 = feedback-in #36(w850) -> ()
            n402 = Increment(x=w828) -> (x+1=→"Scan I (MCL)":u64)
            n403 = To Word Integer(number=w827) -> (16bit integer=w830:i16)
            n404 = Multiply(x=w830, y="Scan freq.  increment (MCL)") -> (x*y=w829:i16)
          }
        }
        n405 = case shown="True" "Multiple trap 3 position offset \nfile" {
          tunnel: ["Piezo Trap Y (AO4)" w812] -> w770
          tunnel: ["Piezo Trap X (AO5)" w811] -> w768
          frame False {
          }
          frame True {
            n406 = local read "Scan I"() -> (w823:u64)
            n407 = Decrement(x=w823) -> (x-1=w824:u64)
            n408 = Quotient & Remainder(x=w824, y="Piezo offset Y points") -> (x-y*floor(x/y)=w821:u64, floor(x/y)=w819:u64)
            n409 = Multiply(x=w821, y="Piezo Offset Increment") -> (x*y=w818:u64)
            n410 = Multiply(x="Piezo Offset Increment", y=w819) -> (x*y=w816:u64)
            n411 = Add(x=w816, y="Piezo offset Xmin") -> (x+y=w813:u64)
            n412 = Add(x=w818, y="Piezo Offset Ymin") -> (x+y=w814:u64)
            n413 = To Word Integer(number=w813) -> (16bit integer=w811:i16)
            n414 = To Word Integer(number=w814) -> (16bit integer=w812:i16)
          }
        }
        n415 = Select(t=w773, s="1D or 2D Scan?", f=i16 0) -> (s? t:f=w774:i16)
        n416 = Select(t=w789, s="MCL Scan Axis", f=w774) -> (s? t:f=w790:i16)
        n417 = Select(t=w774, s="MCL Scan Axis", f=w789) -> (s? t:f=w788:i16)
        n418 = case shown="True" "ScanTrap 3 or Fl-laser" {
          tunnel: w790 -> [w800 w802]
          tunnel: w788 -> [w795 w806]
          tunnel: "AO2 (X)" -> [w796 w807]
          tunnel: "AO1 (Y)" -> [w799 w808]
          tunnel: [w798 w808] -> w778
          tunnel: [w797 w807] -> w777
          tunnel: w770 -> [w794 w803]
          tunnel: [w794 w801] -> w769
          tunnel: w768 -> [w793 w805]
          tunnel: [w793 w804] -> w767
          frame False {
            n419 = Add(x=w796, y=w795) -> (x+y=w797:i16)
            n420 = Add(x=w799, y=w800) -> (x+y=w798:i16)
          }
          frame True {
            n421 = Add(x=w803, y=w802) -> (x+y=w801:i16)
            n422 = Add(x=w805, y=w806) -> (x+y=w804:i16)
          }
        }
      }
      frame #3 {
        n423 = feedback-in #37(w894) -> ()
        n424 = feedback #37(w894) -> (w893:u32)
        n425 = Boolean To (0,1)(Boolean="+ phase (MCL)") -> (0, 1=w885:i16)
        n426 = Subtract(x=w894, y=w893) -> (x-y=w892:u32)
        n427 = Multiply(x=w885, y="Phase count adjustment (MCL)") -> (x*y=w881:i16)
        n428 = Subtract(x=w892, y=w891) -> (x-y=w873:u32)
        n429 = Subtract(x="MCL count", y=w873) -> (x-y=w883:u32)
        n430 = feedback #38(i16 0) -> (w882:i16)
        n431 = Subtract(x=w882, y=w881) -> (x-y=w880:i16)
        "MCL Relative Phase" <- w880
        n432 = feedback-in #38(w880) -> ()
        n433 = Number To Boolean Array(number=w873) -> (Boolean array=w874:bool[])
        n434 = Or Array Elements(Boolean array=w874) -> (logical OR=w872:bool)
        n435 = Boolean To (0,1)(Boolean=w872) -> (0, 1=w879:i16)
        n436 = Add(x=w883, y=w881) -> (x+y=w887:u32)
        n437 = To Unsigned Byte Integer(number=w879) -> (unsigned 8bit integer=w876:u8)
        n438 = feedback #39(u8 0) -> (w877:u8)
        n439 = Add(x=w876, y=w877) -> (x+y=w875:u8)
        "MCL Late Counter" <- w875
        n440 = feedback-in #39(w875) -> ()
        "Piezo Y out" <- w870
        "Piezo X out" <- w869
      }
    }
  }
  n441 = while "Trap RF control, main calculations (raster scanning, intensity and position feedback, phase control etc) with primary timing trigger" {
    shift-right: [w912] -> _
    shift-left: w4 -> [w911]
    shift-right: [w910] -> _
    shift-left: FALSE ("Swap F1 and F2") -> [w909]
    shift-right: [w905] -> _
    shift-left: u16 0 ("BD 1 Amplitude 3") -> [w903]
    shift-right: [w902] -> _
    shift-left: u64 0 -> [w901]
    shift-right: [w900] -> _
    shift-left: u64 0 -> [w898]
    shift-right: [w899] -> _
    shift-left: u64 0 -> [w896]
    stop <- FALSE stop-if-true
    n442 = flat-sequence {
      tunnel: w909 -> [w918]
      tunnel: w911 -> [w916]
      tunnel: [w918] -> w908
      tunnel: [w917] -> w907
      tunnel: [w916] -> w906
      tunnel: [w915] -> w904
      tunnel: w903 -> [w915]
      tunnel: [w914] -> w897
      tunnel: w896 -> [w914]
      tunnel: [w931] -> w912
      tunnel: [w930] -> w910
      tunnel: w908 -> [w929]
      tunnel: w907 -> [w928]
      tunnel: w906 -> [w927]
      tunnel: [w926] -> w905
      tunnel: w904 -> [w925]
      tunnel: [w924] -> w902
      tunnel: w901 -> [w923]
      tunnel: [w922] -> w900
      tunnel: [w921] -> w899
      tunnel: w898 -> [w920]
      tunnel: w897 -> [w919]
      frame #0 {
        n443 = call "Loop Timer"("Count(Ticks)"=w916) -> ("Tick Count(Ticks)"=w917:u16)
      }
      frame #1 {
        n444 = flat-sequence {
          tunnel: w929 -> [w939]
          tunnel: w925 -> [w933]
          tunnel: [w995] -> w931
          tunnel: [w1007] -> w930
          tunnel: w928 -> [w1001]
          tunnel: w927 -> [w998]
          tunnel: [w953] -> w926
          tunnel: [w945] -> w924
          tunnel: w923 -> [w944]
          tunnel: [w943] -> w922
          tunnel: [w942] -> w921
          tunnel: w920 -> [w941]
          tunnel: w919 -> [w940]
          frame #0 {
            w934 = -1 ("Timeout")
            # "Operation when you need a long delay for either X or Y to synchonize AOD light out phase (> ~100 ticks)\nor want shorter trap ON timing. Puts some of the delay timing in parallel with the later computations."
            # "Trigger the external loop by sending the boolean FSK value through a FIFO.\nTiming is precise."
            n445 = Boolean To (0,1)(Boolean=w939) -> (0, 1=w938:i16)
            n446 = To Unsigned Word Integer(number=w938) -> (unsigned 16bit integer=w937:u16)
            n447 = xnode ("FIFO Method Node")("Element"=w937, "Timeout"=w934) -> ("FIFO Out"=w936:refnum<k21>)  [unwired: 1 in, 1 out]
            n448 = xnode ("FIFO Method Node")("Element"=w933, "Timeout"=w934, "FIFO In"=w936) -> ("FIFO Out"=w935:refnum<k21>)  [unwired: 1 out]
            n449 = xnode ("FIFO Method Node")("Element"=i16 0, "Timeout"=w934, "FIFO In"=w935) -> ()  [unwired: 2 out]
          }
          frame #1 {
            # "Just counts, wraps around, 8 bit"
            # "Which trap cycle"
            # "Just flips back and forth."
            # "If interlacing is off, this is which cycle to use."
            # "Keep track of trap cycles (trap 1, 2, 3...)"
            # "This is the prior cycle's on time"
            # "increment timing\nindex, reset to 0 if \nend of matrix"
            # "Reset to begginning (1) when number of cycles reached."
            # "timing index"
            # "build byte stacks for writing data\n(must correspond to addresses array constant)"
            # "Timing housekeeping"
            # "Adjust phase if late\n(maintains constant phase relationship between cycles)"
            n450 = feedback #40(u8 0 ("t")) -> (w1004:u8)
            n451 = Increment(x=w1004) -> (x+1=w1043:u8)
            n452 = Increment(x="Number Interlace Cycles") -> (x+1=w1038:u8)
            n453 = Equal?(x=w1043, y=w1038) -> (x = y?=w1045:bool)
            n454 = Select(t=u8 1, s=w1045, f=w1043) -> (s? t:f=w1003:u8)
            n455 = feedback-in #40(w1003) -> ()
            n456 = Increment(x=w1003) -> (x+1=w1040:u8)
            n457 = Equal?(x=w1040, y=w1038) -> (x = y?=w1041:bool)
            n458 = Select "This cycle"(t=u8 1, s=w1041, f=w1040) -> (s? t:f=w1037:u8)
            n459 = Select(t=w1037, s="Interlace ON/OFF", f="Interlace Off Parameters") -> (s? t:f=w963:u8)
            n460 = feedback-in #41(w1001) -> ()
            n461 = feedback #41(w1001) -> (w1000:u16)
            n462 = Select(t=w1003, s="Interlace ON/OFF", f="Interlace Off Parameters") -> (s? t:f=w1036:u8)
            n463 = Subtract(x=w1001, y=w1000) -> (x-y=w999:u16)
            n464 = Subtract "The error"(x=w999, y=w998) -> (x-y=w982:u16)
            n465 = case shown="1, Default" w1036 {
              tunnel: ["DIO count 1 (ticks)" "DIO count 2 (ticks)" "DIO count 3 (ticks)"] -> w997
              frame 1, Default {
              }
              frame 2 {
              }
              frame 3 {
              }
            }
            n466 = Number To Boolean Array(number=w982) -> (Boolean array=w983:bool[])
            n467 = Or Array Elements(Boolean array=w983) -> (logical OR=w981:bool)
            n468 = Boolean To (0,1)(Boolean=w981) -> (0, 1=w988:i16)
            n469 = To Unsigned Byte Integer(number=w988) -> (unsigned 8bit integer=w985:u8)
            n470 = feedback #42(u8 0) -> (w986:u8)
            n471 = Add(x=w985, y=w986) -> (x+y=w984:u8)
            "DIO Late Counter" <- w984
            n472 = feedback-in #42(w984) -> ()
            n473 = Subtract(x=w997, y=w982) -> (x-y=w996:u16)
            n474 = local read "green FB running"() -> (w970:bool)
            n475 = disable-structure shown="Disabled" {
              disable-tunnel: [w1049 _] -> w980
              disable-tunnel: w963 -> [w1046 _]
              frame Disabled {
                n476 = feedback #43(i64 0 ("y")) -> (w1048:i64)
                n477 = case "Synchronize trap oscillations - always begin/end with trap 1" shown="1, Default" w1046 {
                  tunnel: [w1050 w1051 w1052] -> w1049
                  tunnel: w1048 -> [w1050 w1051 _]
                  frame 2 {
                  }
                  frame 3 {
                  }
                  frame 1, Default {
                    n478 = Or(x="Osc traps", y="Initiate trap osc") -> (x .or. y?=w1054:bool)
                    n479 = case "Trap sine oscillation (or whatever pattern is stored in memory)" shown="True" w1054 {
                      tunnel: [i64 0 ("y") w1058] -> w1052
                      tunnel: "Initiate trap osc" -> [_ w1061]
                      frame False {
                      }
                      frame True {
                        w1065 = u16 0
                        w1063 = -1
                        n480 = local write "Initiate trap osc"(FALSE ("Initiate trap osc")) -> ()
                        n481 = feedback #44(w1065) -> (w1067:u16)
                        n482 = Select(t=w1065, s=w1061, f=w1067) -> (s? t:f=w1066:u16)
                        n483 = Greater Or Equal?(x=w1066, y="Trap osc period (pts)") -> (x >= y?=w1072:bool)
                        n484 = Or(x=w1061, y=w1072) -> (x .or. y?=w1073:bool)
                        n485 = Select(t=u16 0, s=w1073, f=w1066) -> (s? t:f=w1057:u16)
                        n486 = feedback #45(w1063) -> (w1064:i32)
                        n487 = Select(t=w1063, s=w1061, f=w1064) -> (s? t:f=w1062:i32)
                        n488 = Increment(x=w1062) -> (x+1=w1069:i32)
                        n489 = Equal?(x=w1057, y=u16 0) -> (x = y?=w1070:bool)
                        n490 = Increment(x=w1057) -> (x+1=w1077:u16)
                        n491 = feedback-in #44(w1077) -> ()
                        n492 = Select(t=w1069, s=w1070, f=w1062) -> (s? t:f=w1068:i32)
                        n493 = feedback-in #45(w1068) -> ()
                        n494 = case shown="False" "Osc trap cont." {
                          tunnel: w1068 -> [w1081 _]
                          frame False {
                            n495 = Greater Or Equal?(x=w1081, y="N trap osc periods") -> (x >= y?=w1079:bool)
                            n496 = Not(x=w1079) -> (.not. x?=w1078:bool)
                            n497 = local write "Osc traps"(w1078) -> ()
                          }
                          frame True {
                          }
                        }
                        n498 = xnode ("Memory Read")("Address"=w1057, "Memory In"=refnum<k21> "Trap osc memory") -> ("Data"=w1058:i64)  [unwired: 1 out]
                      }
                    }
                  }
                }
                n499 = feedback-in #43(w1049) -> ()
              }
              frame Enabled {
              }
            }
            n500 = And(x=w970, y="RF synth bd controls green") -> (x .and. y?=w969:bool)
            n501 = case shown="1, Default" w963 {
              tunnel: [w1205 w1431 "BD 1 Frequency 3"] -> w1033
              tunnel: [w1252 w1430 w1458] -> w972
              tunnel: [w1202 w1428 "BD 1 Amplitude 3"] -> w953
              tunnel: "FB Gains" -> [w1223 w1437 _]
              tunnel: "FB output range" -> [w1224 w1436 _]
              tunnel: w980 -> [w1221 w1434 _]
              tunnel: "BD 2 Frequency 1" -> [w1218 _ _]
              tunnel: "BD 2 Frequency 2" -> [_ w1430 _]
              tunnel: "BD 2 Frequency 3" -> [_ _ w1458]
              tunnel: w969 -> [_ _ w1457]
              tunnel: [w1205 w1429 w1456] -> w945
              tunnel: w944 -> [w1204 w1429 w1456]
              tunnel: [w1197 u64 0 u64 0] -> w943
              tunnel: [w1198 u64 0 u64 0] -> w942
              tunnel: w941 -> [_ w1424 _]
              tunnel: w940 -> [_ w1423 _]
              frame 1, Default {
                w1238 = fxp<+/-,24,9> 0.0 ("AI1 X Set 2")
                w1232 = u16 0
                w1250 = u64 0 ("f")
                # "#Alex This works with div(Q,R) 2, but I think *2^n is faster, untested"
                # "Changed by RG:\nenables symmetric motion of \ntraps during raster scanning \nand force feedback."
                # "Changed by Ronen - correction \nby PID is now implemented not on \nthe Base BD1 frequency but on the last\nfrequency sent."
                # "Added by Ronen -\nUpper and Lower \nLimits for the FB \ngenerated frequency\nto avoid losing bead \nwhen tether breaks"
                # "Explanation of raster scanning:\n1. Cycles: increment counter by 1 every time interlace cycle returns to trap 1. As long as \n  Cycle per Step is larger than counter, keep incrementing counter and do not change step counter.\n  Once counter is equal to Cycles per step, zero counter and increment step counter.\n2. Steps: Increments up every time cycles counter equals cycles per step. Performs the following:\n- To determine DIRECTION of frequency change:  If ScanstepX2 is EQUAL to step counter (full for-back scan finished)\n   frequency increment is set to zero, AND step counter is set to zero. \n   Otherwise: if no change to step counter (because cycleperstep>cycle counter), then no change to frequency\n   increment. \n   If step counter has changed (cycleperstep=cycle counter), then need to figure out direction of frequency change:\n   if step counter is EQUAL to Scansteps: No change to frequency increment\n   Otherwise: If scan steps > step counter - 1 (forward scan NOT completed): increment frequency by 1\n                       If scan steps equal or smaller than step counter -1 (forward scan completed): increment frequency by -1\n\n3. Scans: Increment scan counter every time step counter equals 2Xscan steps (full for-back scan completed)\n    if number of scans > scan counter: Send TRUE to scanning, continue scan\n    if number of scans = scan counter: Send FALSE to Scanning, Scan finished.\n\n  The wire with the asterik can be used as the index for getting the mirror positions in the offset scan."
                # "This signal integration happens no matter what\nso that correct setpoints can be chosen before \nturning on the FB."
                # "Trap 1"
                n502 = local read "AI1 X Set 2"() -> (w1216:fxp<+/-,16,1>)
                n503 = local read "AI1 X Set 1"() -> (w1235:fxp<+/-,16,1>)
                n504 = local read "Scanning"() -> (w1253:bool)
                n505 = Multiply(x=w1216, y="B factor") -> (x*y=w1214:fxp<+/-,48,17>)
                n506 = Or(x=w1253, y="Start scan") -> (x .or. y?=w1248:bool)
                n507 = case shown="True" "Diff FB Measurement?" {
                  tunnel: w1214 -> [w1278 w1287]
                  tunnel: w1235 -> [w1277 w1288]
                  tunnel: [w1275 w1279] -> w1236
                  frame False {
                    n508 = Select(t=w1277, s="Trap Pos FB Monitor T1 or T2", f=w1278) -> (s? t:f=w1275:fxp<+/-,48,17>)
                  }
                  frame True {
                    n509 = Subtract(x=w1288, y=w1287) -> (x-y=w1280:fxp<+/-,48,17>)
                    n510 = Not(x="Negate Diff?") -> (.not. x?=w1286:bool)
                    n511 = Boolean To (0,1)(Boolean="Negate Diff?") -> (0, 1=w1284:i16)
                    n512 = Boolean To (0,1)(Boolean=w1286) -> (0, 1=w1285:i16)
                    n513 = Negate(x=w1284) -> (-x=w1283:i16)
                    n514 = Add(x=w1283, y=w1285) -> (x+y=w1281:i16)
                    n515 = Multiply(x=w1281, y=w1280) -> (x*y=w1279:fxp<+/-,63,32>)
                  }
                }
                n516 = Not(x="Abort scan") -> (.not. x?=w1246:bool)
                n517 = And(x=w1246, y=w1248) -> (x .and. y?=w1245:bool)
                n518 = case "For raster scanning" shown="False" w1245 {
                  tunnel: [i64 0 w1411] -> w1200
                  tunnel: "Start scan" -> [_ w1396]
                  tunnel: [u64 1 w1373] -> w1217
                  frame False {
                    n519 = local write "Scanning"(FALSE ("scanning")) -> ()
                  }
                  frame True {
                    w1380 = i64 0
                    w1379 = u64 0
                    # "scan incr."
                    # "freq. incr. mult."
                    # "count steps"
                    # "count number of cycles"
                    n520 = feedback #46(w1379) -> (w1408:u64)
                    n521 = Select(t=w1379, s=w1396, f=w1408) -> (s? t:f=w1410:u64)
                    n522 = Increment(x=w1410) -> (x+1=w1407:u64)
                    n523 = Greater?(x="Cycles per step", y=w1407) -> (0:w1389:bool)
                    n524 = Select(t=w1407, s=w1389, f=w1379) -> (s? t:f=w1406:u64)
                    n525 = feedback-in #46(w1406) -> ()
                    n526 = feedback #47(w1379) -> (w1405:u64)
                    n527 = Select(t=w1379, s=w1396, f=w1405) -> (s? t:f=w1400:u64)
                    n528 = Increment(x=w1400) -> (x+1=w1404:u64)
                    n529 = Add(x="Scan steps", y="Scan steps") -> (x+y=w1403:u64)
                    n530 = Select(t=w1400, s=w1389, f=w1404) -> (s? t:f=w1384:u64)
                    n531 = Greater?(x=w1403, y=w1384) -> (0:w1383:bool)
                    n532 = Select(t=w1384, s=w1383, f=w1379) -> (s? t:f=w1401:u64)
                    n533 = feedback-in #47(w1401) -> ()
                    n534 = Equal?(x="Scan steps", y=w1384) -> (x = y?=w1388:bool)
                    n535 = Greater?(x="Scan steps", y=w1400) -> (0:w1399:bool)
                    n536 = feedback #48(w1380) -> (w1402:i64)
                    n537 = Select(t=w1380, s=w1396, f=w1402) -> (s? t:f=w1386:i64)
                    n538 = Increment(x=w1386) -> (x+1=w1398:i64)
                    n539 = Decrement(x=w1386) -> (x-1=w1397:i64)
                    n540 = Select(t=w1398, s=w1399, f=w1397) -> (s? t:f=w1387:i64)
                    n541 = Select(t=w1386, s=w1388, f=w1387) -> (s? t:f=w1385:i64)
                    n542 = Select(t=w1386, s=w1389, f=w1385) -> (s? t:f=w1381:i64)
                    n543 = Select(t=w1381, s=w1383, f=w1380) -> (s? t:f=w1382:i64)
                    n544 = feedback-in #48(w1382) -> ()
                    n545 = feedback #49(w1379) -> (w1395:u64)
                    n546 = Select(t=w1379, s=w1396, f=w1395) -> (s? t:f=w1391:u64)
                    n547 = Increment(x=w1391) -> (x+1=w1392:u64)
                    n548 = Select(t=w1391, s=w1383, f=w1392) -> (s? t:f=w1390:u64)
                    n549 = Greater?(x="Number of scans", y=w1390) -> (0:w1376:bool)
                    n550 = Multiply(x="Scan freq.  increment", y=w1386) -> (x*y=w1411:i64)
                    n551 = Select(t=TRUE, s="Cont. Scan", f=w1376) -> (s? t:f=w1375:bool)
                    "Scanning" <- w1375
                    n552 = Select(t=w1390, s=w1375, f=w1379) -> (s? t:f=w1393:u64)
                    n553 = feedback-in #49(w1393) -> ()
                    n554 = Increment(x=w1390) -> (x+1=w1373:u64)
                  }
                }
                "Scan I" <- w1217
                n555 = feedback #50(w1232) -> (w1231:u16)
                n556 = Increment(x=w1231) -> (x+1=w1233:u16)
                n557 = Greater Or Equal?(x=w1233, y="Trap Pos FB Int Count") -> (x >= y?=w1203:bool)
                n558 = Select(t=w1232, s=w1203, f=w1233) -> (s? t:f=w1234:u16)
                n559 = feedback-in #50(w1234) -> ()
                n560 = feedback #51(w1238) -> (w1237:fxp<+/-,24,9>)
                n561 = Add(x=w1236, y=w1237) -> (x+y=w1230:fxp<+/-,24,9>)
                n562 = case "Trap 1 X intensity feedback" shown="True" "FB On/Off Set 1" {
                  tunnel: "BD 1 Amplitude 1" -> [w1413 _]
                  tunnel: [w1413 w1417] -> w1202
                  tunnel: w1224 -> [_ w1414]
                  tunnel: w1223 -> [_ w1415]
                  frame False {
                  }
                  frame True {
                    n563 = local read "AI2 Y Sum Set 1"() -> (w1418:i16)
                    n564 = call "Slower PID.vi"("process variable"=w1418, "reset?"="FB Reset Set 1", "setpoint"="FB Setpoint Set 1", "PID gains (x 2^8)"=w1415, "output range"=w1414) -> ("output"=w1419:i16)  [unwired: 10 out]
                    n565 = To Unsigned Word Integer(number=w1419) -> (unsigned 16bit integer=w1417:u16)
                  }
                }
                "BD1 amplitude 1 out" <- w1202
                n566 = Select(t=w1238, s=w1203, f=w1230) -> (s? t:f=w1241:fxp<+/-,24,9>)
                n567 = feedback-in #51(w1241) -> ()
                n568 = Divide(x=w1230, y="Trap Pos FB Int Count") -> (x/y=w1225:fxp<+/-,16,1>)
                n569 = feedback #52(fxp<+/-,24,9> 0.0 ("AI1 X Set 2")) -> (w1242:fxp<+/-,24,9>)
                n570 = Select(t=w1230, s=w1203, f=w1242) -> (s? t:f=w1243:fxp<+/-,24,9>)
                "Trap Pos FB Int Signal" <- w1243
                n571 = feedback-in #52(w1243) -> ()
                n572 = feedback #53(fxp<+/-,16,1> 0.0 ("Trap Pos FB Int-Norm Signal")) -> (w1227:fxp<+/-,16,1>)
                n573 = Select(t=w1225, s=w1203, f=w1227) -> (s? t:f=w1226:fxp<+/-,16,1>)
                "Trap Pos FB Int-Norm Signal" <- w1226
                n574 = feedback-in #53(w1226) -> ()
                n575 = case "For position feedback" shown="True" "Force feedback" {
                  tunnel: [i64 0 w1294] -> w1199
                  tunnel: w1225 -> [_ w1291]
                  tunnel: w1203 -> [_ w1290]
                  frame False {
                  }
                  frame True {
                    n576 = feedback #54(i64 0) -> (w1293:i64)
                    n577 = case shown="True" w1290 {
                      tunnel: [w1295 w1299] -> w1294
                      tunnel: w1293 -> [w1295 _]
                      tunnel: w1291 -> [_ w1298]
                      frame False {
                      }
                      frame True {
                        n578 = xnode ("PID")("process variable"=w1298, "reset?"="Trap Pos. FB Reset", "setpoint"="Trap Pos. FB SP", "PID gains"="Trap Pos. FB Gains", "output range"="Trap pos. FB Range") -> ("output"=w1308:fxp<+/-,16,1>)
                        n579 = Negate(x=w1308) -> (-x=w1307:fxp<+/-,17,2>)
                        n580 = Select(t=w1307, s="Trap Pos FB Negate Action", f=w1308) -> (s? t:f=w1304:fxp<+/-,17,2>)
                        n581 = Scale By Power Of 2(n=u32 15, x=u32 1) -> (x*2^n=w1301:u32)
                        n582 = Multiply(x=w1304, y=w1301) -> (x*y=w1300:fxp<+/-,17,17>)
                        n583 = To Quad Integer(1:w1300) -> (0:w1312:i64)
                        "Trap Pos FB Action" <- w1312
                        n584 = Multiply(x=w1312, y="Trap Pos. FB Mult Factor") -> (x*y=w1310:i64)
                        n585 = Add(x=w1310, y="Trap Pos. FB Offset Factor") -> (x+y=w1299:i64)
                        n586 = disable-structure shown="Disabled" {
                          disable-tunnel: w1299 -> [w1319 _]
                          frame Disabled {
                            w1323 = u32 0
                            n587 = feedback #55() -> (w1320:i64)  [unwired: 1 in]
                            n588 = Add(x=w1319, y=w1320) -> (x+y=w1317:i64)
                            n589 = feedback #56(w1323) -> (w1325:u32)
                            n590 = Increment(x=w1325) -> (x+1=w1314:u32)
                            n591 = Greater Or Equal?(x=w1314, y="FB Trig Integrate") -> (x >= y?=w1315:bool)
                            n592 = Select(t=i64 0, s=w1315, f=w1317) -> (s? t:f=w1321:i64)
                            n593 = feedback-in #55(w1321) -> ()
                            n594 = Select(t=w1323, s=w1315, f=w1314) -> (s? t:f=w1324:u32)
                            n595 = feedback-in #56(w1324) -> ()
                            n596 = And(x=w1315, y="FPGA Trap Trig") -> (x .and. y?=w1322:bool)
                            n597 = case "Trap FB trigger excitation laser ON" shown="True" w1322 {
                              tunnel: w1317 -> [_ w1329]
                              tunnel: w1314 -> [_ w1327]
                              frame False {
                              }
                              frame True {
                                n598 = Not(x="TTrig Negate Pos") -> (.not. x?=w1336:bool)
                                n599 = Boolean To (0,1)(Boolean="TTrig Negate Pos") -> (0, 1=w1334:i16)
                                n600 = Boolean To (0,1)(Boolean=w1336) -> (0, 1=w1335:i16)
                                n601 = Negate(x=w1334) -> (-x=w1333:i16)
                                n602 = Add(x=w1333, y=w1335) -> (x+y=w1332:i16)
                                n603 = Multiply(x=w1332, y=w1329) -> (x*y=w1331:i64)
                                "TTrig Sig" <- w1331
                                n604 = Multiply(x="FPGA TTrig Thresh", y=w1327) -> (x*y=w1328:i64)
                                "TTrig Fin Thresh" <- w1328
                                n605 = Greater Or Equal?(x=w1331, y=w1328) -> (x >= y?=w1330:bool)
                                n606 = case shown="True" w1330 {
                                frame False {
                                }
                                frame True {
                                w1339 = TRUE ("Green FB On/Off")
                                w1341 = u8 2 ("Operating Mode")
                                n607 = local write "Operating Mode 2"(w1341) -> ()
                                n608 = local write "Operating Mode"(w1341) -> ()
                                n609 = local write "Green FB On/Off"(w1339) -> ()
                                n610 = local write "FPGA Trap Trig"(FALSE ("FPGA Trap Trig")) -> ()
                                "TTrig?" <- w1339
                                }
                                }
                              }
                            }
                          }
                          frame Enabled {
                          }
                        }
                      }
                    }
                    n611 = feedback-in #54(w1294) -> ()
                  }
                }
                n612 = case shown="True" "Symmetric force feedback\nand raster scan" {
                  tunnel: [w1257 w1260] -> w1197
                  tunnel: w1200 -> [w1257 w1261]
                  tunnel: [w1256 w1258] -> w1198
                  tunnel: w1199 -> [w1256 w1259]
                  frame False {
                  }
                  frame True {
                    n613 = Scale By Power Of 2(n=i16 -1, x=w1261) -> (x*2^n=w1260:i64)
                    n614 = Scale By Power Of 2(n=i16 -1, x=w1259) -> (x*2^n=w1258:i64)
                  }
                }
                n615 = And(x="Force feedback", y="Dynamic Force FB (Ronen)") -> (x .and. y?=w1211:bool)
                n616 = case shown="False" w1211 {
                  tunnel: w1198 -> [w1266 w1270]
                  tunnel: [w1265 w1269] -> w1210
                  tunnel: w1204 -> [_ w1268]
                  tunnel: w1203 -> [_ w1267]
                  frame False {
                    # "(BD1 Frequency 1)"
                    n617 = Add(x="BD 1 Frequency 1", y=w1266) -> (x+y=w1265:u64)
                  }
                  frame True {
                    n618 = case shown="True" w1267 {
                      tunnel: w1270 -> [_ w1274]
                      tunnel: [w1271 w1273] -> w1269
                      tunnel: w1268 -> [w1271 w1272]
                      frame False {
                      }
                      frame True {
                        n619 = Add(x=w1272, y=w1274) -> (x+y=w1273:u64)
                      }
                    }
                  }
                }
                n620 = Select(t=w1221, s="Trap 1 osc enable", f=i64 0) -> (s? t:f=w1219:i64)
                n621 = Select(t=w1250, s="Scan BD", f=w1197) -> (s? t:f=w1249:u64)
                n622 = Select(t=w1197, s="Scan BD", f=w1250) -> (s? t:f=w1209:u64)
                n623 = Add(x=w1249, y=w1218) -> (x+y=w1252:u64)
                n624 = Compound Arithmetic op=ADD(w1219, w1210, w1209) -> (w1208:u64)
                n625 = In Range and Coerce(upper limit="FB Max Frequency", x=w1208, lower limit="FB Min frequency") -> (coerced(x)=w1205:u64)  [unwired: 1 out]
                "BD1 Frequency Out 1" <- w1205
              }
              frame 2 {
                # "Trap 2"
                n626 = local read "Symmetric force feedback\nand raster scan"() -> (w1427:bool)
                n627 = case shown="True" w1427 {
                  tunnel: "BD 1 Frequency 2" -> [w1440 w1445]
                  tunnel: [w1440 w1441] -> w1425
                  tunnel: w1424 -> [_ w1444]
                  tunnel: w1423 -> [_ w1442]
                  frame False {
                  }
                  frame True {
                    n628 = Subtract(x=w1445, y=w1444) -> (x-y=w1443:u64)
                    n629 = Subtract(x=w1443, y=w1442) -> (x-y=w1441:u64)
                  }
                }
                n630 = case "Trap 2 X intensity feedback" shown="True" "FB On/Off Set 2" {
                  tunnel: [w1446 w1449] -> w1428
                  tunnel: "BD 1 Amplitude 2" -> [w1446 _]
                  tunnel: w1437 -> [_ w1448]
                  tunnel: w1436 -> [_ w1447]
                  frame False {
                  }
                  frame True {
                    n631 = local read "AI2 Y Sum Set 2"() -> (w1452:i16)
                    n632 = call "Slower PID.vi"("process variable"=w1452, "reset?"="FB Reset Set 2", "setpoint"="FB Setpoint Set 2", "PID gains (x 2^8)"=w1448, "output range"=w1447) -> ("output"=w1450:i16)  [unwired: 10 out]
                    n633 = To Unsigned Word Integer(number=w1450) -> (unsigned 16bit integer=w1449:u16)
                  }
                }
                "BD1 amplitude 2 out" <- w1428
                n634 = Select(t=w1434, s="Trap 2 osc enable", f=i64 0) -> (s? t:f=w1433:i64)
                n635 = Add(x=w1425, y=w1433) -> (x+y=w1431:u64)
                "BD1 Frequency Out 2" <- w1431
              }
              frame 3 {
                # "Fluorescence period"
                n636 = disable-structure shown="Disabled" {
                  disable-tunnel: [w1466 _] -> _
                  disable-tunnel: w1457 -> [w1465 _]
                  frame Disabled {
                    # "Remember if FB was previously on/off"
                    n637 = feedback #57(FALSE) -> (w1461:bool)
                    n638 = case shown="True" w1465 {
                      tunnel: [w1468 w1484] -> w1466
                      tunnel: "BD 2 Amplitude 3" -> [w1468 _]
                      tunnel: [FALSE TRUE] -> w1462
                      tunnel: w1461 -> [_ w1469]
                      frame False {
                      }
                      frame True {
                        # "Makes it so first time FB run when turned on, the PID sees the detector intensity from the last time FB was running, rather than something near zero. Especially assuming the setpoint is not changing, this will make the FB more stable when resuming, and not overshoot the turnon intensity."
                        # "FB output range: 0 should be low, full scale is 12 bits.\nBut be careful not to go over, then higher bits just get ignored by RF board, so output will actually jump down and be unstable. Keep it under 4000 to be safe."
                        n639 = local read "Green FB Sum"() -> (w1472:i16)
                        n640 = feedback-in #58(w1472) -> ()
                        n641 = feedback #58(i16 0 ("Green FB Sum")) -> (w1471:i16)
                        n642 = Select(t=w1472, s=w1469, f=w1471) -> (s? t:f=w1470:i16)
                        n643 = Bundle("P3 2"="P3 2", "I3 2"="I3 2", "D3 2"="D3 2") -> (w1483:cluster{"P3 2":i16, "I3 2":i16, "D3 2":i16})  [unwired: 1 in]
                        n644 = Bundle("RF synth green feedback max"="RF synth green feedback max", i16 0) -> (w1475:cluster{"RF synth green feedback max":i16, i16})  [unwired: 1 in]
                        n645 = call "Slower PID.vi"("process variable"=w1470, "reset?"="Green FB Reset 2", "setpoint"="Green FB Setpoint 2", "PID gains (x 2^8)"=w1483, "output range"=w1475) -> ("output"=w1485:i16)  [unwired: 10 out]
                        n646 = To Unsigned Word Integer(number=w1485) -> (unsigned 16bit integer=w1484:u16)
                      }
                    }
                    n647 = feedback-in #57(w1462) -> ()
                  }
                  frame Enabled {
                  }
                }
              }
            }
            n648 = Split Number(x=w1033) -> (hi(x)=w1032:u32, lo(x)=w1031:u32)
            n649 = Boolean To (0,1)(Boolean="+ phase (DIO)") -> (0, 1=w993:i16)
            n650 = Split Number(x=w1032) -> (lo(x)=w1030:u16)  [unwired: 1 out]
            n651 = Split Number(x=w1031) -> (hi(x)=w1029:u16, lo(x)=w1028:u16)
            n652 = Split Number(x=w1030) -> (hi(x)=w1022:u8, lo(x)=w1021:u8)
            n653 = Split Number(x=w1029) -> (hi(x)=w1020:u8, lo(x)=w1019:u8)
            n654 = Split Number(x=w1028) -> (hi(x)=w1018:u8, lo(x)=w1017:u8)
            n655 = Multiply(x=w993, y="Phase count adjustment (DIO)") -> (x*y=w989:i16)
            n656 = feedback #59(TRUE) -> (w978:bool)
            n657 = Not(x=w978) -> (.not. x?=w977:bool)
            n658 = feedback-in #59(w977) -> ()
            n659 = feedback #60(i16 0) -> (w991:i16)
            n660 = Subtract(x=w991, y=w989) -> (x-y=w990:i16)
            "DIO Relative phase" <- w990
            n661 = feedback-in #60(w990) -> ()
            n662 = Add(x=w996, y=w989) -> (x+y=w995:u16)
            n663 = Build Array "BD 1 nu Stack"(w1022, w1021, w1020, w1019, w1018, w1017) -> (w1016:u8[])
            n664 = case "Store in RF board F1 or F2" shown="True" w977 {
              tunnel: [w1188 w1192] -> w1007
              tunnel: [u8 10 u8 4] -> w1008
              tunnel: "Swap F1 and F2" -> [w1189 w1192]
              tunnel: "BD 2 Frequency 1" -> [_ w1191]
              tunnel: "BD 2 Frequency 2" -> [w1187 _]
              tunnel: [w1187 w1191] -> w973
              frame False {
                # "for RF synth controls\ngreen: F1/F2 stay same"
                # "F2 address (hex)"
                n665 = Not(x=w1189) -> (.not. x?=w1188:bool)
              }
              frame True {
                # "low chooses F1"
                # "F1 address (hex)"
              }
            }
            n666 = Select(t=w973, s="RF synth bd controls green", f=w972) -> (s? t:f=w971:u64)
            n667 = Split Number(x=w971) -> (hi(x)=w1027:u32, lo(x)=w1026:u32)
            n668 = Split Number(x=w1027) -> (lo(x)=w1025:u16)  [unwired: 1 out]
            n669 = Split Number(x=w1026) -> (hi(x)=w1024:u16, lo(x)=w1023:u16)
            n670 = Split Number(x=w1025) -> (hi(x)=w1015:u8, lo(x)=w1014:u8)
            n671 = Split Number(x=w1024) -> (hi(x)=w1013:u8, lo(x)=w1012:u8)
            n672 = Split Number(x=w1023) -> (hi(x)=w1011:u8, lo(x)=w1010:u8)
            n673 = Build Array "BD 2 nu Stack"(w1015, w1014, w1013, w1012, w1011, w1010) -> (w1009:u8[])
            n674 = flat-sequence "Update trap RF synth board settings to be used for the upcoming trap cycle." {
              tunnel: w1009 -> [w1136]
              tunnel: w1016 -> [w1137]
              tunnel: [w1137] -> w967
              tunnel: [w1136] -> w966
              tunnel: w1008 -> [w1138]
              tunnel: w967 -> [w1140]
              tunnel: w966 -> [w1139]
              tunnel: w954 -> [w1151]
              tunnel: w956 -> [w1150]
              tunnel: w955 -> [w1149]
              frame #0 {
                # "To possibly delay\nthese writes to very\nend of loop (for x and\ny phase adjust)"
                n675 = call "Wait8"("Count(Ticks)"="Next trap write delay (ticks)") -> ()  [unwired: 1 out]
              }
              frame #1 {
                # "Next trap RF frequency:\n\nWrite next trap cycle frequency to buffer."
                n676 = for {
                  tunnel: w1140 -> [w1146] mode=indexing
                  tunnel: w1139 -> [w1145] mode=indexing
                  tunnel: w1138 -> [w1143]
                  i -> [w1144]
                  n677 = To Unsigned Byte Integer(number=w1144) -> (unsigned 8bit integer=w1141:u8)
                  n678 = Add(x=w1143, y=w1141) -> (x+y=w1142:u8)
                  n679 = call "write to RF synth bd.vi"("Address Byte"=w1142, "BD 2 Byte"=w1145, "BD 1 Byte"=w1146) -> ()
                }
              }
              frame #2 {
                w1147 = TRUE ("Connector1/DIO15")
                # "Send udclk high\n(BD 1 and 2) to make the new frequency active in F1 or F2 word. But it won't actually be the used frequency until FSK switches to it (begining of next cycle)."
                n680 = xnode "FPGA I/O Node"("Connector1/DIO30"=w1147, "Connector1/DIO29"=w1147) -> ()  [unwired: 2 in, 2 out]
              }
              frame #3 {
                w1148 = FALSE ("Connector1/DIO15")
                n681 = xnode "FPGA I/O Node"("Connector1/DIO30"=w1148, "Connector1/DIO29"=w1148) -> ()  [unwired: 2 in, 2 out]
              }
              frame #4 {
                # "Next trap RF phase offset:\n\nSet the next trap cycle amplitude to the buffer. Won't become active until udclk is set high at proper time at the begining of the next cycle."
                n682 = case shown="True" w1151 {
                  tunnel: w1150 -> [_ w1152]
                  tunnel: w1149 -> [_ w1153]
                  frame False {
                  }
                  frame True {
                    # "phase 1 address start"
                    n683 = for {
                      tunnel: w1152 -> [w1160] mode=indexing
                      tunnel: w1153 -> [w1159] mode=indexing
                      tunnel: u8 0 -> [w1157]
                      i -> [w1158]
                      n684 = To Unsigned Byte Integer(number=w1158) -> (unsigned 8bit integer=w1155:u8)
                      n685 = Add(x=w1157, y=w1155) -> (x+y=w1156:u8)
                      n686 = call "write to RF synth bd.vi"("Address Byte"=w1156, "BD 2 Byte"=w1159, "BD 1 Byte"=w1160) -> ()
                    }
                  }
                }
              }
              frame #5 {
                # "Prep to reset RF phase to zero at start of next cycle. Only reset BD 1. Do nothing to BD 2. This puts the settings in the buffer. A udclk high will make both this phase reset and possibly a new phase offset setting active."
                n687 = case shown="True" "RF phase reset before cycles" {
                  frame False {
                  }
                  frame True {
                    w1163 = u8 66  # BD 1 reset
                    n688 = call "write to RF synth bd.vi"("Address Byte"=u8 31, "BD 2 Byte"=u8 2, "BD 1 Byte"=w1163) -> ()
                  }
                }
              }
              frame #6 {
                # "Address"
                # "Data BD 2"
                # "Data BD 1"
                # "If phase reset wasn't chosen previously, these actions will have no affect. For both BD's, data should be binary 10, and address should be hex 1F (bin 01 1111)"
                # "This sets up the digital communication lines to restart phase accumulation (start RF running agin). It cancels out the possible phase reset. Just need to set WR DIO low then udclk DIOhigh  to make this happen. Doing this here early (and not using the usual board write function) speeds things up.\n\nRestarts RF (BD 1 only, BD2 never stopped in first place)."
                n689 = xnode "FPGA I/O Node"("Connector1/DIO0"=FALSE, "Connector1/DIO1"=FALSE, "Connector1/DIO2"=FALSE, "Connector1/DIO3"=FALSE, "Connector1/DIO4"=FALSE, "Connector1/DIO5"=FALSE, "Connector1/DIO6"=TRUE, "Connector1/DIO7"=FALSE, "Connector1/DIO8"=FALSE, "Connector1/DIO9"=TRUE, "Connector1/DIO10"=TRUE, "Connector1/DIO11"=TRUE, "Connector1/DIO12"=TRUE, "Connector1/DIO13"=TRUE, "Connector1/DIO20"=FALSE, "Connector1/DIO21"=FALSE, "Connector1/DIO22"=FALSE, "Connector1/DIO23"=FALSE, "Connector1/DIO24"=FALSE, "Connector1/DIO25"=FALSE, "Connector1/DIO26"=TRUE, "Connector1/DIO27"=FALSE) -> ()  [unwired: 22 in, 22 out]
              }
            }
            n690 = feedback #61(fxp<+,8,8> 0.0) -> (w950:fxp<+,8,8>)
            n691 = Increment(x=w950) -> (x+1=w948:fxp<+,8,8>)
            n692 = feedback-in #61(w948) -> ()
            n693 = case "Trap RF phase offset control methods" shown="3" "Phase offset method" {
              tunnel: [fxp<+,14,14> 0.0 ("Phase BD 1") w1086 w1101 w1130] -> w957
              tunnel: "Phase Trap 1" -> [_ w1087 w1102 _]
              tunnel: w963 -> [_ w1088 w1103 w1131]
              tunnel: [FALSE TRUE TRUE TRUE] -> w954
              tunnel: "Phase Trap 2" -> [_ w1084 w1099 _]
              tunnel: w948 -> [_ _ w1098 _]
              frame 0, Default {
              }
              frame 1 {
                # "Constant increment of phase offset with each trap cycle. This results in a constant phase difference between trap cycles. \nOnly for traps 1 and 2 (set phase offset to zero for set three)."
                n694 = case shown="1, Default" w1088 {
                  tunnel: w1087 -> [_ _ w1094]
                  tunnel: [w1090 fxp<+,14,14> 0.0 w1095] -> w1086
                  tunnel: w1084 -> [w1089 _ _]
                  frame 2 {
                    n695 = feedback #62(fxp<+,14,14> 0.0) -> (w1092:fxp<+,14,14>)
                    n696 = Add(x=w1089, y=w1092) -> (x+y=w1090:fxp<+,14,14>)
                    n697 = feedback-in #62(w1090) -> ()
                  }
                  frame 3 {
                  }
                  frame 1, Default {
                    n698 = feedback #63(fxp<+,14,14> 0.0) -> (w1097:fxp<+,14,14>)
                    n699 = Add(x=w1094, y=w1097) -> (x+y=w1095:fxp<+,14,14>)
                    n700 = feedback-in #63(w1095) -> ()
                  }
                }
              }
              frame 2 {
                # "Changing increment of phase offset with each trap cycle. This results in a constant change in phase difference between trap cycles. \nOnly for traps 1 and 2 (set phase offset to zero for set three)."
                n701 = case shown="2" w1103 {
                  tunnel: w1102 -> [_ _ w1113]
                  tunnel: [w1104 fxp<+,14,14> 0.0 w1111] -> w1101
                  tunnel: w1099 -> [w1106 _ _]
                  tunnel: w1098 -> [w1107 _ w1114]
                  frame 2 {
                    n702 = Multiply(x=w1106, y=w1107) -> (x*y=w1105:fxp<+,16,16>)
                    n703 = feedback #64(fxp<+,14,14> 0.0) -> (w1109:fxp<+,14,14>)
                    n704 = Add(x=w1105, y=w1109) -> (x+y=w1104:fxp<+,14,14>)
                    n705 = feedback-in #64(w1104) -> ()
                  }
                  frame 3 {
                  }
                  frame 1, Default {
                    n706 = Multiply(x=w1113, y=w1114) -> (x*y=w1112:fxp<+,16,16>)
                    n707 = feedback #65(fxp<+,14,14> 0.0) -> (w1116:fxp<+,14,14>)
                    n708 = Add(x=w1112, y=w1116) -> (x+y=w1111:fxp<+,14,14>)
                    n709 = feedback-in #65(w1111) -> ()
                  }
                }
              }
              frame 3 {
                w1123 = u32 1013904223  # LCG constant C (add)
                w1125 = fxp<+,21,21> 1664525.0  # LCG constant A (multiply)
                # "Set a random phase offset. Random number generated using the LCG method. Constants and method taken from NI white noise generator code (method is general though)."
                # "shift to 14 significant bits"
                n710 = feedback #66(u32 4294967295 ("seed")) -> (w1120:u32)
                n711 = Multiply(x=w1120, y=w1125) -> (x*y=w1124:u32)
                n712 = Split Number(x=w1120) -> (hi(x)=w1126:u16)  [unwired: 1 out]
                n713 = To Unsigned Word Integer(number=w1126) -> (unsigned 16bit integer=w1118:u16)
                n714 = Add(x=w1124, y=w1123) -> (x+y=w1122:fxp<+,32,32>)
                n715 = To Unsigned Long Integer(number=w1122) -> (unsigned 32bit integer=w1119:u32)
                n716 = feedback-in #66(w1119) -> ()
                n717 = Scale By Power Of 2(n=i8 -2 ("Uniform scale factor"), x=w1118) -> (x*2^n=w1127:u16)
                n718 = To Fixed-Point(number=w1127) -> (fixed-point=w1117:fxp<+,14,14>)  [unwired: 1 in]
                "Random phase generated" <- w1117
                n719 = case shown="1, Default" w1131 {
                  tunnel: [w1132 fxp<+,14,14> 0.0 w1134] -> w1130
                  tunnel: w1117 -> [w1132 _ w1134]
                  frame 2 {
                  }
                  frame 3 {
                  }
                  frame 1, Default {
                  }
                }
              }
            }
            n720 = To Unsigned Word Integer(number=w957) -> (unsigned 16bit integer=w962:u16)
            n721 = Split Number(x=w962) -> (hi(x)=w960:u8, lo(x)=w961:u8)
            n722 = Split Number(x=u16 0) -> (hi(x)=w958:u8, lo(x)=w959:u8)
            n723 = Build Array ("BD 1 A Stack")(w960, w961) -> (w956:u8[])
            n724 = Build Array ("BD 1 A Stack")(w958, w959) -> (w955:u8[])
          }
        }
      }
    }
  }
  n725 = while "RF synth board interlacing timing loop" {
    tunnel: w4 -> [_]
    stop <- FALSE stop-if-true
    # "This loop is stalled until the RF FIFO get a value. With this method we gain additional delay time (because  we allow the rest of the main RF loop to procede while this loop waits to send the switch signals - a form of parallelism). This helps to simplify the main RF code. \n\nThe code also allow optimal interlacing while also controlling trap RF phase. \n\nNote: a lot of work has gone into optimizing these methods and it is unclear how they can be made any faster or better than this (many failed tries). Right now there is essentially ~4 ticks (~90 ns ns) of imperfection in the switching from trap 1 to trap 2. ~2 ticks of no RF (phase reset) then ~2 ticks of trap 2 with the wrong amplitude (T1 amplitude). The total ticks is 200, so not a big error.\n\nPhase can be precisely set for each trap. Phase reset and switching, has similar delays as fsk frequency switching. And phase reset and phase offset changes are also not simultaneous. So we can't perfectly line everything up.\n\nIf you start from amp zero though (as for trap 1), the on switch is perfect. Likewise the off is perfect for trap 2. \n\nThe green laser switching is also perfect because of its reduced duty cycle and delays in fsk switching between 80 and 0 MHz."
    n726 = xnode ("FIFO Read")("Timeout"=-1) -> ("Element"=w1532:u16, "FIFO Out"=w1528:refnum<k21>)  [unwired: 1 in, 1 out]
    n727 = Equal To 0?(x=w1532) -> (x = 0?=w1529:bool)
    n728 = Not(x=w1529) -> (.not. x?=w1486:bool)
    n729 = flat-sequence "BD 1 and 2 RF phase and amplitude switching" {
      tunnel: w1486 -> [_]
      tunnel: w1521 -> [w1636]
      tunnel: w1520 -> [w1635]
      tunnel: w1519 -> [w1634]
      tunnel: w1518 -> [w1633]
      tunnel: w1517 -> [w1632]
      tunnel: w1516 -> [w1631]
      tunnel: w1515 -> [w1630]
      tunnel: w1514 -> [w1629]
      tunnel: w1512 -> [w1628]
      tunnel: w1511 -> [w1627]
      tunnel: w1510 -> [w1626]
      tunnel: w1508 -> [w1624]
      tunnel: w1507 -> [w1623]
      tunnel: w1506 -> [w1622]
      tunnel: w1509 -> [w1625]
      tunnel: w1513 -> [w1621]
      tunnel: w1505 -> [w1660]
      tunnel: w1504 -> [w1659]
      tunnel: w1503 -> [w1658]
      tunnel: w1502 -> [w1657]
      tunnel: w1501 -> [w1656]
      tunnel: w1500 -> [w1655]
      tunnel: w1499 -> [w1654]
      tunnel: w1498 -> [w1653]
      tunnel: w1497 -> [w1652]
      tunnel: w1495 -> [w1651]
      tunnel: w1494 -> [w1650]
      tunnel: w1493 -> [w1649]
      tunnel: w1492 -> [w1648]
      tunnel: w1491 -> [w1647]
      tunnel: w1490 -> [w1646]
      tunnel: w1496 -> [w1645]
      frame #0 {
        # "Delay to align amp/frequency switching depending on the method used.\n\nCan also give enough time to do the parallel amplitude calculations"
        n730 = call "Wait"("Count(Ticks)"="Amp switch delay") -> ()  [unwired: 1 out]
      }
      frame #1 {
        w1616 = TRUE ("Connector1/DIO30")
        # "make phase offset and phase reset active with buffer transfer"
        n731 = xnode "FPGA I/O Node"("Connector1/DIO29"=w1616, "Connector1/DIO30"=w1616) -> ()  [unwired: 2 in, 2 out]
      }
      frame #2 {
        w1617 = FALSE ("Connector1/DIO15")
        # "write phase restart to buffer and reset udclk"
        n732 = xnode "FPGA I/O Node"("Connector1/DIO29"=w1617, "Connector1/DIO30"=w1617, "Connector1/DIO15"=FALSE ("Connector1/DIO14")) -> ()  [unwired: 3 in, 3 out]
      }
      frame #3 {
        w1619 = TRUE ("Connector1/DIO15")
        # "make phase restart active"
        # "reset WR"
        n733 = xnode "FPGA I/O Node"("Connector1/DIO15"=w1619, "Connector1/DIO29"=w1619, "Connector1/DIO30"=w1619) -> ()  [unwired: 3 in, 3 out]
      }
      frame #4 {
        w1620 = FALSE ("Connector1/DIO30")
        # "Address"
        # "set amp byte 1, and reset udclk"
        n734 = xnode "FPGA I/O Node"("Connector1/DIO0"=w1636, "Connector1/DIO1"=w1635, "Connector1/DIO2"=w1634, "Connector1/DIO3"=w1633, "Connector1/DIO4"=w1632, "Connector1/DIO5"=w1631, "Connector1/DIO6"=w1630, "Connector1/DIO7"=w1629, "Connector1/DIO8"=TRUE, "Connector1/DIO9"=FALSE, "Connector1/DIO10"=FALSE, "Connector1/DIO11"=FALSE, "Connector1/DIO12"=FALSE, "Connector1/DIO13"=TRUE, "Connector1/DIO20"=w1621, "Connector1/DIO21"=w1628, "Connector1/DIO22"=w1627, "Connector1/DIO23"=w1626, "Connector1/DIO24"=w1625, "Connector1/DIO25"=w1624, "Connector1/DIO26"=w1623, "Connector1/DIO27"=w1622, "Connector1/DIO30"=w1620, "Connector1/DIO29"=w1620) -> ()  [unwired: 24 in, 24 out]
      }
      frame #5 {
        # "write amp byte 1 to buffer"
        n735 = xnode "FPGA I/O Node"("Connector1/DIO15"=FALSE ("Connector1/DIO14")) -> ()  [unwired: 1 in, 1 out]
      }
      frame #6 {
        # "reset WR"
        n736 = xnode "FPGA I/O Node"("Connector1/DIO15"=TRUE) -> ()  [unwired: 1 in, 1 out]
      }
      frame #7 {
        # "Address"
        # "set amp byte 2"
        n737 = xnode "FPGA I/O Node"("Connector1/DIO0"=w1660, "Connector1/DIO1"=w1659, "Connector1/DIO2"=w1658, "Connector1/DIO3"=w1657, "Connector1/DIO4"=w1656, "Connector1/DIO5"=w1655, "Connector1/DIO6"=w1654, "Connector1/DIO7"=w1653, "Connector1/DIO8"=TRUE, "Connector1/DIO9"=FALSE, "Connector1/DIO10"=FALSE, "Connector1/DIO11"=FALSE, "Connector1/DIO12"=TRUE, "Connector1/DIO13"=FALSE, "Connector1/DIO20"=w1652, "Connector1/DIO21"=w1645, "Connector1/DIO22"=w1651, "Connector1/DIO23"=w1650, "Connector1/DIO24"=w1649, "Connector1/DIO25"=w1648, "Connector1/DIO26"=w1647, "Connector1/DIO27"=w1646) -> ()  [unwired: 22 in, 22 out]
      }
      frame #8 {
        # "write amp byte 2"
        n738 = xnode "FPGA I/O Node"("Connector1/DIO15"=FALSE ("Connector1/DIO14")) -> ()  [unwired: 1 in, 1 out]
      }
      frame #9 {
        w1668 = TRUE ("Connector1/DIO15")
        # "transfer amp bytes 1 and 2 and reset WR"
        n739 = xnode "FPGA I/O Node"("Connector1/DIO29"=w1668, "Connector1/DIO30"=w1668, "Connector1/DIO15"=TRUE ("Connector1/DIO14")) -> ()  [unwired: 3 in, 3 out]
      }
      frame #10 {
        w1670 = FALSE ("Connector1/DIO14")
        # "reset udclk"
        n740 = xnode "FPGA I/O Node"("Connector1/DIO29"=w1670, "Connector1/DIO30"=w1670) -> ()  [unwired: 2 in, 2 out]
      }
    }
    n741 = flat-sequence "FSK BD 1 (trap X)" {
      tunnel: w1486 -> [w1534]
      tunnel: [w1534] -> w1489
      tunnel: w1489 -> [w1535]
      frame #0 {
        n742 = call "Wait2"("Count(Ticks)"="BD 1 Delay (ticks)") -> ()  [unwired: 1 out]
      }
      frame #1 {
        # "switch frequency"
        n743 = xnode "FPGA I/O Node"("Connector1/DIO36"=w1535) -> ()  [unwired: 1 in, 1 out]
      }
    }
    n744 = flat-sequence "FSK BD 2 (trap Y or green laser AOM)" {
      tunnel: w1486 -> [w1672]
      tunnel: [w1672] -> w1531
      tunnel: w1531 -> [w1673]
      frame #0 {
        n745 = call "Wait11"("Count(Ticks)"="BD 2 Delay (Ticks)") -> ()  [unwired: 1 out]
      }
      frame #1 {
        # "switch frequency"
        n746 = xnode "FPGA I/O Node"("Connector1/DIO37"=w1673) -> ()  [unwired: 1 in, 1 out]
      }
    }
    n747 = xnode ("FIFO Read")("Timeout"=-1, "FIFO In"=w1528) -> ("Element"=w1523:u16, "FIFO Out"=w1527:refnum<k21>)  [unwired: 1 out]
    n748 = xnode ("FIFO Read")("Timeout"=-1, "FIFO In"=w1527) -> ("Element"=w1522:u16)  [unwired: 2 out]
    n749 = node-c288() -> (w1525:T6)  [unwired: 1 in]
    n750 = timed-loop "Convert amplitude words to bits" {
      timing: w1525 -> [_]
      timing-out: [_] -> w1524
      tunnel: w1523 -> [w1592]
      tunnel: w1522 -> [w1591]
      tunnel: [w1568] -> w1521
      tunnel: [w1567] -> w1520
      tunnel: [w1566] -> w1519
      tunnel: [w1565] -> w1518
      tunnel: [w1564] -> w1517
      tunnel: [w1563] -> w1516
      tunnel: [w1562] -> w1515
      tunnel: [w1561] -> w1514
      tunnel: [w1560] -> w1513
      tunnel: [w1559] -> w1512
      tunnel: [w1558] -> w1511
      tunnel: [w1557] -> w1510
      tunnel: [w1556] -> w1509
      tunnel: [w1555] -> w1508
      tunnel: [w1554] -> w1507
      tunnel: [w1553] -> w1506
      tunnel: [w1552] -> w1505
      tunnel: [w1551] -> w1504
      tunnel: [w1550] -> w1503
      tunnel: [w1549] -> w1502
      tunnel: [w1548] -> w1501
      tunnel: [w1547] -> w1500
      tunnel: [w1546] -> w1499
      tunnel: [w1545] -> w1498
      tunnel: [w1544] -> w1497
      tunnel: [w1543] -> w1496
      tunnel: [w1542] -> w1495
      tunnel: [w1541] -> w1494
      tunnel: [w1540] -> w1493
      tunnel: [w1539] -> w1492
      tunnel: [w1538] -> w1491
      tunnel: [w1537] -> w1490
      stop <- TRUE stop-if-true
      # "Board 1 Data"
      # "Board 2 Data"
      # "Board 1 Data"
      # "Board 2 Data"
      n751 = Split Number(x=w1592) -> (hi(x)=w1590:u8, lo(x)=w1570:u8)
      n752 = Split Number(x=w1591) -> (hi(x)=w1589:u8, lo(x)=w1569:u8)
      n753 = Number To Boolean Array(number=w1590) -> (Boolean array=w1610:bool[])
      n754 = Number To Boolean Array(number=w1589) -> (Boolean array=w1601:bool[])
      n755 = Index Array(array=w1610, index=7) -> (element=w1568:bool)
      n756 = Index Array(array=w1610, index=6) -> (element=w1567:bool)
      n757 = Index Array(array=w1610, index=5) -> (element=w1566:bool)
      n758 = Index Array(array=w1610, index=4) -> (element=w1565:bool)
      n759 = Index Array(array=w1610, index=3) -> (element=w1564:bool)
      n760 = Index Array(array=w1610, index=2) -> (element=w1563:bool)
      n761 = Index Array(array=w1610, index=1) -> (element=w1562:bool)
      n762 = Index Array(array=w1610, index=0) -> (element=w1561:bool)
      n763 = Index Array(array=w1601, index=7) -> (element=w1560:bool)
      n764 = Index Array(array=w1601, index=6) -> (element=w1559:bool)
      n765 = Index Array(array=w1601, index=5) -> (element=w1558:bool)
      n766 = Index Array(array=w1601, index=4) -> (element=w1557:bool)
      n767 = Index Array(array=w1601, index=3) -> (element=w1556:bool)
      n768 = Index Array(array=w1601, index=2) -> (element=w1555:bool)
      n769 = Index Array(array=w1601, index=1) -> (element=w1554:bool)
      n770 = Index Array(array=w1601, index=0) -> (element=w1553:bool)
      n771 = Number To Boolean Array(number=w1570) -> (Boolean array=w1588:bool[])
      n772 = Number To Boolean Array(number=w1569) -> (Boolean array=w1579:bool[])
      n773 = Index Array(array=w1588, index=7) -> (element=w1552:bool)
      n774 = Index Array(array=w1588, index=6) -> (element=w1551:bool)
      n775 = Index Array(array=w1588, index=5) -> (element=w1550:bool)
      n776 = Index Array(array=w1588, index=4) -> (element=w1549:bool)
      n777 = Index Array(array=w1588, index=3) -> (element=w1548:bool)
      n778 = Index Array(array=w1588, index=2) -> (element=w1547:bool)
      n779 = Index Array(array=w1588, index=1) -> (element=w1546:bool)
      n780 = Index Array(array=w1588, index=0) -> (element=w1545:bool)
      n781 = Index Array(array=w1579, index=7) -> (element=w1544:bool)
      n782 = Index Array(array=w1579, index=6) -> (element=w1543:bool)
      n783 = Index Array(array=w1579, index=5) -> (element=w1542:bool)
      n784 = Index Array(array=w1579, index=4) -> (element=w1541:bool)
      n785 = Index Array(array=w1579, index=3) -> (element=w1540:bool)
      n786 = Index Array(array=w1579, index=2) -> (element=w1539:bool)
      n787 = Index Array(array=w1579, index=1) -> (element=w1538:bool)
      n788 = Index Array(array=w1579, index=0) -> (element=w1537:bool)
    }
    n789 = node-c288(w1524) -> ()
  }
  n790 = while "Control APD data integration - stream to host" {
    shift-right: [w1677] -> _
    shift-left: w3 -> [w1682]
    stop <- FALSE stop-if-true
    n791 = flat-sequence {
      tunnel: w1682 -> [w1684]
      tunnel: [w1685] -> w1680
      tunnel: [w1684] -> w1678
      tunnel: [w1695] -> w1681
      tunnel: w1680 -> [w1695]
      tunnel: [w1694] -> w1679
      tunnel: w1678 -> [w1694]
      tunnel: [w1693] -> w1676
      tunnel: [w1692] -> w1675
      tunnel: [w1686] -> w1674
      tunnel: [w1743] -> w1677
      tunnel: w1681 -> [w1752]
      tunnel: w1679 -> [w1749]
      tunnel: w1676 -> [w1736]
      tunnel: w1675 -> [w1735]
      tunnel: w1674 -> [w1723]
      frame #0 {
        n792 = call "Loop Timer6"("Count(Ticks)"=w1684) -> ("Tick Count(Ticks)"=w1685:u32)
      }
      frame #1 {
        n793 = flat-sequence {
          tunnel: [w1697] -> w1691
          tunnel: w1691 -> [w1701]
          tunnel: [w1703] -> w1690
          tunnel: [w1702] -> w1689
          tunnel: [w1701] -> w1688
          tunnel: [i16 0] -> w1687
          tunnel: [w1714] -> w1692
          tunnel: [w1715] -> w1693
          tunnel: w1690 -> [w1715]
          tunnel: w1689 -> [w1714]
          tunnel: w1688 -> [w1713]
          tunnel: w1687 -> [w1712]
          tunnel: [w1712] -> w1686
          frame #0 {
            # "use separate variable so each APD won't\nhave to wait to read"
            n794 = feedback #67(FALSE) -> (w1696:bool)
            "APD1 out state" <- w1696
            "APD2 out state" <- w1696
            n795 = disable-structure shown="Disabled" {
              disable-tunnel: w1696 -> [w1699 _]
              frame Disabled {
                "APD3 out state" <- w1699
              }
              frame Enabled {
              }
            }
            n796 = Not(x=w1696) -> (.not. x?=w1697:bool)
            n797 = feedback-in #67(w1697) -> ()
          }
          frame #1 {
            n798 = disable-structure shown="Disabled" {
              disable-tunnel: w1701 -> [w1709 _]
              disable-tunnel: [w1708 _] -> _
              frame Disabled {
                n799 = local read "APD 3 Counts 1"() -> (w1711:u32)
                n800 = local read "APD 3 Counts 0"() -> (w1710:u32)
                n801 = Select(t=w1711, s=w1709, f=w1710) -> (s? t:f=w1708:u32)
              }
              frame Enabled {
              }
            }
            n802 = local read "APD 1 Counts 1"() -> (w1707:u32)
            n803 = local read "APD 1 Counts 0"() -> (w1706:u32)
            n804 = local read "APD 2 Counts 1"() -> (w1705:u32)
            n805 = local read "APD 2 Counts 0"() -> (w1704:u32)
            n806 = Select(t=w1707, s=w1701, f=w1706) -> (s? t:f=w1703:u32)
            n807 = Select(t=w1705, s=w1701, f=w1704) -> (s? t:f=w1702:u32)
          }
          frame #2 {
            n808 = case shown="True" w1713 {
              frame False {
                w1716 = u32 0 ("APD 1 Counts 0")
                n809 = disable-structure shown="Disabled" {
                  disable-tunnel: w1716 -> [w1717 _]
                  frame Disabled {
                    n810 = local write "APD 3 Counts 0"(w1717) -> ()
                  }
                  frame Enabled {
                  }
                }
                n811 = local write "APD 1 Counts 0"(w1716) -> ()
                n812 = local write "APD 2 Counts 0"(w1716) -> ()
              }
              frame True {
                w1718 = u32 0 ("APD 1 Counts 1")
                n813 = disable-structure shown="Disabled" {
                  disable-tunnel: w1718 -> [w1719 _]
                  frame Disabled {
                    n814 = local write "APD 3 Counts 1"(w1719) -> ()
                  }
                  frame Enabled {
                  }
                }
                n815 = local write "APD 1 Counts 1"(w1718) -> ()
                n816 = local write "APD 2 Counts 1"(w1718) -> ()
              }
            }
          }
        }
      }
      frame #2 {
        # "crude initialization: if APD to FIFO is off (usually\nonly before initializing a measurement) count is forced to 0\nand green to true"
        # "count cycles till switching"
        n817 = feedback-in #68(w1752) -> ()
        n818 = feedback #68(w1752) -> (w1751:u32)
        n819 = Subtract(x=w1752, y=w1751) -> (x-y=w1750:u32)
        n820 = Subtract(x=w1750, y=w1749) -> (x-y=w1728:u32)
        n821 = case shown="True" "APD to FIFO" {
          tunnel: w1736 -> [_ w1757]
          tunnel: w1735 -> [_ w1755]
          tunnel: w1723 -> [_ w1753]
          frame False {
          }
          frame True {
            n822 = flat-sequence {
              tunnel: 0 ("Timeout") -> [w1759]
              tunnel: w1757 -> [w1760]
              tunnel: [w1759] -> w1756
              tunnel: w1756 -> [w1761]
              tunnel: w1755 -> [w1762]
              tunnel: [w1761] -> w1754
              tunnel: w1754 -> [w1764]
              tunnel: w1753 -> [w1763]
              frame #0 {
                n823 = xnode ("FIFO Write")("Element"=w1760, "Timeout"=w1759) -> ()  [unwired: 1 in, 2 out]
              }
              frame #1 {
                n824 = xnode ("FIFO Write")("Element"=w1762, "Timeout"=w1761) -> ()  [unwired: 1 in, 2 out]
              }
              frame #2 {
                n825 = xnode ("FIFO Write")("Element"=w1763, "Timeout"=w1764) -> ()  [unwired: 1 in, 2 out]
              }
            }
          }
        }
        n826 = Subtract(x="APD Acq Rate Count", y=w1728) -> (x-y=w1744:u32)
        n827 = Number To Boolean Array(number=w1728) -> (Boolean array=w1729:bool[])
        n828 = Or Array Elements(Boolean array=w1729) -> (logical OR=w1727:bool)
        n829 = Boolean To (0,1)(Boolean=w1727) -> (0, 1=w1734:i16)
        n830 = To Unsigned Byte Integer(number=w1734) -> (unsigned 8bit integer=w1731:u8)
        n831 = feedback #69(u8 0) -> (w1732:u8)
        n832 = Add(x=w1731, y=w1732) -> (x+y=w1730:u8)
        "APD Acq Late Counter" <- w1730
        n833 = feedback-in #69(w1730) -> ()
        n834 = Boolean To (0,1)(Boolean="+ phase (APD Acq)") -> (0, 1=w1740:i16)
        n835 = Multiply(x=w1740, y="Phase Count Adjustment (APD Acq)") -> (x*y=w1737:i16)
        n836 = Add(x=w1744, y=w1737) -> (x+y=w1743:u32)
        n837 = feedback #70(i16 0) -> (w1742:i16)
        n838 = Subtract(x=w1742, y=w1737) -> (x-y=w1739:i16)
        "APD Acq Relative Phase" <- w1739
        n839 = feedback-in #70(w1739) -> ()
        n840 = To Word Integer(number=w1736) -> (16bit integer=w1745:i16)
        n841 = To Word Integer(number=w1723) -> (16bit integer=w1724:i16)
        n842 = To Word Integer(number=w1735) -> (16bit integer=w1746:i16)
        n843 = Multiply(x="APD AO scale factor", y=w1746) -> (x*y=w1725:i16)
        n844 = Multiply(x="APD AO scale factor", y=w1724) -> (x*y=w1721:i16)
        n845 = Multiply(x="APD AO scale factor", y=w1745) -> (x*y=w1726:i16)
        n846 = xnode "FPGA I/O Node"("Connector0/AO5"=w1726, "Connector0/AO7"=w1725, "Connector0/AO6"=w1721) -> ()  [unwired: 3 in, 3 out]
      }
    }
  }
  n847 = disable-structure shown="Disabled" {
    disable-tunnel: w4 -> [w1765 _]
    frame Disabled {
      n848 = while "APD 3 Counter" {
        tunnel: w1765 -> [_]
        stop <- FALSE stop-if-true
        n849 = flat-sequence {
          frame #0 {
            n850 = xnode "FPGA I/O Method Node"("FPGA I/O In"=refnum<k21> "Connector0/DIO12" ("APD 2 DO"), "Timeout"=-1) -> ()  [unwired: 2 out]
          }
          frame #1 {
            n851 = local read "APD3 int gate"() -> (w1769:bool)
            n852 = case shown="True" w1769 {
              frame False {
              }
              frame True {
                n853 = local read "APD3 out state"() -> (w1770:bool)
                n854 = case shown="True" w1770 {
                  frame False {
                    n855 = local read "APD 3 Counts 0"() -> (w1772:u32)
                    n856 = Increment(x=w1772) -> (x+1=→"APD 3 Counts 0":u32)
                  }
                  frame True {
                    n857 = local read "APD 3 Counts 1"() -> (w1774:u32)
                    n858 = Increment(x=w1774) -> (x+1=→"APD 3 Counts 1":u32)
                  }
                }
              }
            }
          }
        }
      }
    }
    frame Enabled {
    }
  }
  n859 = disable-structure shown="Disabled" {
    disable-tunnel: w4 -> [w1776 _]
    disable-tunnel: w5 -> [w1775 _]
    frame Disabled {
      n860 = while "APD 3 Gating" {
        shift-right: [w1780] -> _
        shift-left: w1776 -> [w1785]
        shift-right: [w1779] -> _
        shift-left: w1775 -> [w1777]
        stop <- FALSE stop-if-true
        n861 = flat-sequence {
          tunnel: w1785 -> [w1788]
          tunnel: [w1789] -> w1783
          tunnel: [w1788] -> w1781
          tunnel: [w1787] -> w1778
          tunnel: w1777 -> [w1787]
          tunnel: [w1792] -> w1784
          tunnel: w1783 -> [w1792]
          tunnel: [w1791] -> w1782
          tunnel: w1781 -> [w1791]
          tunnel: w1778 -> [w1790]
          tunnel: [w1813] -> w1780
          tunnel: w1784 -> [w1824]
          tunnel: w1782 -> [w1821]
          tunnel: [w1793] -> w1779
          frame #0 {
            n862 = call "Loop Timer15"("Count(Ticks)"=w1788) -> ("Tick Count(Ticks)"=w1789:u16)
          }
          frame #1 {
            # "Signal maybe then sent through \na transistor before APD"
            n863 = xnode "FPGA I/O Node"("Connector0/DIO2"=w1790) -> ()  [unwired: 1 in, 1 out]
            "APD3 int gate" <- w1790
          }
          frame #2 {
            n864 = local read "APD Gate OFF Count"() -> (w1798:u16)
            n865 = local read "APD Gate ON Count"() -> (w1799:u16)
            n866 = feedback #71(TRUE) -> (w1818:bool)
            n867 = feedback-in #72(w1824) -> ()
            n868 = feedback #72(w1824) -> (w1823:u16)
            n869 = Not(x=w1818) -> (.not. x?=w1816:bool)
            n870 = feedback-in #71(w1816) -> ()
            n871 = Subtract(x=w1824, y=w1823) -> (x-y=w1822:u16)
            n872 = Select(t=w1799, s=w1816, f=w1798) -> (s? t:f=w1820:u16)
            n873 = Subtract(x=w1822, y=w1821) -> (x-y=w1801:u16)
            n874 = Subtract(x=w1820, y=w1801) -> (x-y=w1812:u16)
            n875 = Number To Boolean Array(number=w1801) -> (Boolean array=w1802:bool[])
            n876 = Or Array Elements(Boolean array=w1802) -> (logical OR=w1800:bool)
            n877 = Boolean To (0,1)(Boolean=w1800) -> (0, 1=w1807:i16)
            n878 = Boolean To (0,1)(Boolean="+ phase (APD 3 Gate)") -> (0, 1=w1810:i16)
            n879 = To Unsigned Byte Integer(number=w1807) -> (unsigned 8bit integer=w1804:u8)
            n880 = Multiply(x=w1810, y="Phase count adjustment (APD 3 Gate)") -> (x*y=w1808:i16)
            n881 = feedback #73(u8 0) -> (w1805:u8)
            n882 = Add(x=w1804, y=w1805) -> (x+y=w1803:u8)
            "APD 3 Gate Late Counter" <- w1803
            n883 = feedback-in #73(w1803) -> ()
            n884 = Add(x=w1812, y=w1808) -> (x+y=w1813:u16)
            n885 = feedback #74(i16 0) -> (w1815:i16)
            n886 = Subtract(x=w1815, y=w1808) -> (x-y=w1814:i16)
            "APD 3 Gate Relative Phase" <- w1814
            n887 = feedback-in #74(w1814) -> ()
            n888 = local read "APD Gate Operating Mode"() -> (w1797:u8)
            n889 = case shown="2" w1797 {
              tunnel: [TRUE FALSE w1827] -> w1794
              tunnel: w1818 -> [_ _ w1827]
              frame 0, Default {
              }
              frame 1 {
              }
              frame 2 {
              }
            }
            n890 = local read "Invert APD Gate"() -> (w1796:bool)
            n891 = Not(x=w1794) -> (.not. x?=w1795:bool)
            n892 = Select(t=w1795, s=w1796, f=w1794) -> (s? t:f=w1793:bool)
          }
        }
      }
    }
    frame Enabled {
    }
  }
  n893 = while {
    shift-right: [w1830] -> _
    shift-left: w4 -> [w1836]
    shift-right: [w1831] -> _
    shift-left: _ -> [w1828]
    stop <- FALSE stop-if-true
    n894 = flat-sequence {
      tunnel: w1836 -> [w1839]
      tunnel: [w1840] -> w1834
      tunnel: [w1839] -> w1832
      tunnel: [w1838] -> w1829
      tunnel: w1828 -> [w1838]
      tunnel: [w1843] -> w1835
      tunnel: w1834 -> [w1843]
      tunnel: [w1842] -> w1833
      tunnel: w1832 -> [w1842]
      tunnel: w1829 -> [w1841]
      tunnel: w1835 -> [w1873]
      tunnel: w1833 -> [w1872]
      tunnel: [w1845] -> w1831
      tunnel: [w1844] -> w1830
      frame #0 {
        n895 = call "Loop Timer2"("Count(Ticks)"=w1839) -> ("Tick Count(Ticks)"=w1840:u16)
      }
      frame #1 {
        n896 = xnode "FPGA I/O Node"("Connector0/DIO10"=w1841) -> ()  [unwired: 1 in, 1 out]
      }
      frame #2 {
        n897 = feedback #75(w1873) -> (w1874:u16)
        n898 = feedback-in #75(w1873) -> ()
        n899 = Subtract(x=w1873, y=w1874) -> (x-y=w1875:u16)
        n900 = Subtract(x=w1875, y=w1872) -> (x-y=w1865:u16)
        n901 = Number To Boolean Array(number=w1865) -> (Boolean array=w1870:bool[])
        n902 = Or Array Elements(Boolean array=w1870) -> (logical OR=w1871:bool)
        n903 = Boolean To (0,1)(Boolean="+ phase (EMCCD Gate)") -> (0, 1=w1858:i16)
        n904 = Boolean To (0,1)(Boolean=w1871) -> (0, 1=w1866:i16)
        n905 = To Unsigned Byte Integer(number=w1866) -> (unsigned 8bit integer=w1869:u8)
        n906 = Multiply(x=w1858, y="Phase Count Adjustment EMCCD Gate") -> (x*y=w1860:i16)
        n907 = feedback #76(u8 0) -> (w1868:u8)
        n908 = Add(x=w1869, y=w1868) -> (x+y=w1864:u8)
        "EMCCD Late counter" <- w1864
        n909 = feedback-in #76(w1864) -> ()
        n910 = feedback #77(i16 0) -> (w1859:i16)
        n911 = Subtract(x=w1859, y=w1860) -> (x-y=w1853:i16)
        "EMCCD relative phase" <- w1853
        n912 = feedback-in #77(w1853) -> ()
        n913 = feedback #78(TRUE) -> (w1851:bool)
        n914 = Not(x=w1851) -> (.not. x?=w1849:bool)
        n915 = Select(t="EMCCD Gate ON count", s=w1849, f="EMCCD Gate OFF count") -> (s? t:f=w1861:u16)
        n916 = Subtract(x=w1861, y=w1865) -> (x-y=w1854:u16)
        n917 = Add(x=w1854, y=w1860) -> (x+y=w1844:u16)
        n918 = feedback-in #78(w1849) -> ()
        n919 = case shown="1" "EMCCD Gate Operating Mode" {
          tunnel: w1849 -> [_ _ w1878]
          tunnel: [TRUE FALSE w1878] -> w1847
          frame 0, Default {
          }
          frame 1 {
          }
          frame 2 {
          }
        }
        n920 = Not(x=w1847) -> (.not. x?=w1848:bool)
        n921 = Select(t=w1848, s="Invert EMCCD Gate", f=w1847) -> (s? t:f=w1845:bool)
      }
    }
  }
  n922 = disable-structure shown="Disabled" {
    disable-tunnel: w4 -> [w1881 _]
    disable-tunnel: w15 -> [w1880 _]
    frame Disabled {
      n923 = while "633 nm red  fluorescent laser interlacing (DO to IA 633 nm AOM ME amp)." {
        shift-right: [w2002] -> _
        shift-left: w1881 -> [w2007]
        shift-right: [w2001] -> _
        shift-left: w1880 -> [w1999]
        stop <- FALSE stop-if-true
        n924 = flat-sequence {
          tunnel: w2007 -> [w2010]
          tunnel: [w2011] -> w2005
          tunnel: [w2010] -> w2003
          tunnel: [w2009] -> w2000
          tunnel: w1999 -> [w2009]
          tunnel: [w2014] -> w2006
          tunnel: w2005 -> [w2014]
          tunnel: [w2013] -> w2004
          tunnel: w2003 -> [w2013]
          tunnel: w2000 -> [w2012]
          tunnel: [w2023] -> w2002
          tunnel: w2006 -> [w2043]
          tunnel: w2004 -> [w2040]
          tunnel: [w2032] -> w2001
          frame #0 {
            n925 = call "Loop Timer11"("Count(Ticks)"=w2010) -> ("Tick Count(Ticks)"=w2011:u16)
          }
          frame #1 {
            # "Then to PRL 440 amp"
            n926 = xnode "FPGA I/O Node"("Connector1/DIO32"=w2012) -> ()  [unwired: 1 in, 1 out]
          }
          frame #2 {
            n927 = feedback-in #79(w2043) -> ()
            n928 = feedback #79(w2043) -> (w2042:u16)
            n929 = Subtract(x=w2043, y=w2042) -> (x-y=w2041:u16)
            n930 = Subtract(x=w2041, y=w2040) -> (x-y=w2016:u16)
            n931 = Number To Boolean Array(number=w2016) -> (Boolean array=w2017:bool[])
            n932 = Or Array Elements(Boolean array=w2017) -> (logical OR=w2015:bool)
            n933 = Boolean To (0,1)(Boolean="+ phase (RI)") -> (0, 1=w2028:i16)
            n934 = Multiply(x=w2028, y="Phase count adjustment (RI)") -> (x*y=w2025:i16)
            n935 = Boolean To (0,1)(Boolean=w2015) -> (0, 1=w2022:i16)
            n936 = To Unsigned Byte Integer(number=w2022) -> (unsigned 8bit integer=w2019:u8)
            n937 = feedback #80(i16 0) -> (w2026:i16)
            n938 = feedback #81(u8 0) -> (w2020:u8)
            n939 = Add(x=w2019, y=w2020) -> (x+y=w2018:u8)
            "RI Late Counter" <- w2018
            n940 = feedback-in #81(w2018) -> ()
            n941 = Subtract(x=w2026, y=w2025) -> (x-y=w2024:i16)
            "RI Relative phase" <- w2024
            n942 = feedback-in #80(w2024) -> ()
            n943 = feedback #82(TRUE) -> (w2035:bool)
            n944 = case shown="2" "Red Laser Operating Mode" {
              tunnel: [TRUE FALSE w2049] -> w2032
              tunnel: w2035 -> [_ _ w2046]
              frame 0, Default {
              }
              frame 1 {
              }
              frame 2 {
                n945 = Not(x=w2046) -> (.not. x?=w2048:bool)
                n946 = Select(t=w2048, s="Invert RI", f=w2046) -> (s? t:f=w2049:bool)
              }
            }
            n947 = Not(x=w2035) -> (.not. x?=w2031:bool)
            n948 = Select(t="Red interlace ON count", s=w2031, f="Red interlace OFF count") -> (s? t:f=w2037:u16)
            n949 = Subtract(x=w2037, y=w2016) -> (x-y=w2029:u16)
            n950 = Add(x=w2029, y=w2025) -> (x+y=w2023:u16)
            n951 = feedback-in #82(w2031) -> ()
          }
        }
      }
      n952 = while "473 nm blue  fluorescent laser interlacing (DO to blue laser digital control input)." {
        shift-right: [w1898] -> _
        shift-left: w1881 -> [w1901]
        shift-right: [w1897] -> _
        shift-left: w1880 -> [w1895]
        shift-right: [w1890] -> _
        shift-left: _ -> [w1889]
        shift-right: [w1882] -> _
        shift-left: u16 0 -> [w1885]
        stop <- FALSE stop-if-true
        n953 = flat-sequence {
          tunnel: w1901 -> [w1906]
          tunnel: [w1907] -> w1900
          tunnel: [w1906] -> w1899
          tunnel: [w1905] -> w1896
          tunnel: w1895 -> [w1905]
          tunnel: w1889 -> [w1904]
          tunnel: [w1904] -> w1888
          tunnel: [w1903] -> w1886
          tunnel: w1885 -> [w1903]
          tunnel: [w1912] -> w1894
          tunnel: w1900 -> [w1912]
          tunnel: [w1911] -> w1893
          tunnel: w1899 -> [w1911]
          tunnel: w1896 -> [w1910]
          tunnel: w1888 -> [w1909]
          tunnel: [w1909] -> w1887
          tunnel: w1886 -> [w1908]
          tunnel: [w1908] -> w1884
          tunnel: [w1917] -> w1892
          tunnel: [w1916] -> w1891
          tunnel: w1893 -> [w1916]
          tunnel: w1894 -> [w1917]
          tunnel: w1887 -> [w1915]
          tunnel: w1884 -> [w1914]
          tunnel: [w1913] -> w1883
          tunnel: [w1974] -> w1898
          tunnel: w1892 -> [w1992]
          tunnel: w1891 -> [w1989]
          tunnel: [w1962] -> w1897
          tunnel: [w1960] -> w1890
          tunnel: w1883 -> [w1957]
          tunnel: [w1958] -> w1882
          frame #0 {
            n954 = call "Loop Timer14"("Count(Ticks)"=w1906) -> ("Tick Count(Ticks)"=w1907:u16)
          }
          frame #1 {
            n955 = xnode "FPGA I/O Node"("Connector1/DIO28"=w1910) -> ()  [unwired: 1 in, 1 out]
          }
          frame #2 {
            n956 = case shown="True" w1915 {
              tunnel: w1914 -> [w1918 w1920]
              tunnel: [w1918 w1919] -> w1913
              frame False {
              }
              frame True {
                n957 = flat-sequence {
                  tunnel: [w1926] -> w1923
                  tunnel: [w1925] -> w1922
                  tunnel: [w1924] -> w1921
                  tunnel: w1920 -> [w1924]
                  tunnel: w1923 -> [w1943]
                  tunnel: w1922 -> [w1940]
                  tunnel: w1921 -> [w1942]
                  tunnel: [w1941] -> w1919
                  frame #0 {
                    # "5 ns timing resolution"
                    n958 = node-c288() -> (w1929:T6)  [unwired: 1 in]
                    n959 = timed-loop {
                      timing: w1929 -> [_]
                      timing-out: [_] -> w1928
                      tunnel: "Lifetime timeout APD1" -> [w1935]
                      tunnel: [w1930] -> w1925
                      tunnel: [w1931] -> w1926
                      i -> [w1932]
                      stop <- w1934 stop-if-true
                      n960 = xnode "FPGA I/O Node"() -> ("Connector0/DIO5"=w1933:bool)  [unwired: 1 in, 1 out]
                      n961 = To Unsigned Word Integer(number=w1932) -> (unsigned 16bit integer=w1930:u16)
                      n962 = Equal?(x=w1935, y=w1930) -> (x = y?=w1931:bool)
                      n963 = Or(x=w1933, y=w1931) -> (x .or. y?=w1934:bool)
                    }
                    n964 = node-c288(w1928) -> ()
                  }
                  frame #1 {
                    n965 = Not(x=w1943) -> (.not. x?=w1944:bool)
                    n966 = case shown="True" w1944 {
                      tunnel: w1940 -> [_ w1946]
                      tunnel: w1942 -> [w1945 w1948]
                      tunnel: [w1945 w1947] -> w1941
                      frame False {
                        # "timed out, do nothing"
                      }
                      frame True {
                        # "photon detected,record time"
                        n967 = case shown="True" "Lifetime to FIFO" {
                          tunnel: w1946 -> [_ w1954]
                          tunnel: w1948 -> [w1950 w1952]
                          tunnel: [w1950 w1951] -> w1947
                          frame False {
                            # "don't record time\n(can't if doing force feedback)"
                          }
                          frame True {
                            # "number of events in fifo"
                            n968 = xnode ("FIFO Method Node")("Element"=w1954, "Timeout"=0) -> ()  [unwired: 1 in, 2 out]
                            n969 = Increment(x=w1952) -> (x+1=w1951:u16)
                          }
                        }
                        "lifetime (ticks)" <- w1946
                      }
                    }
                  }
                }
              }
            }
          }
          frame #3 {
            # "Reading fifo is tricky here since\nunknown # of events"
            # "For lifetime measurement:\nInterlacing and pulse falling"
            n970 = feedback-in #83(w1992) -> ()
            n971 = feedback #83(w1992) -> (w1991:u16)
            n972 = Subtract(x=w1992, y=w1991) -> (x-y=w1990:u16)
            n973 = Subtract(x=w1990, y=w1989) -> (x-y=w1967:u16)
            n974 = Number To Boolean Array(number=w1967) -> (Boolean array=w1968:bool[])
            n975 = Or Array Elements(Boolean array=w1968) -> (logical OR=w1966:bool)
            n976 = Boolean To (0,1)(Boolean="+ phase (BI D)") -> (0, 1=w1979:i16)
            n977 = Multiply(x=w1979, y="Phase count adjustment (BI D)") -> (x*y=w1976:i16)
            n978 = Boolean To (0,1)(Boolean=w1966) -> (0, 1=w1973:i16)
            n979 = To Unsigned Byte Integer(number=w1973) -> (unsigned 8bit integer=w1970:u8)
            n980 = feedback #84(i16 0) -> (w1977:i16)
            n981 = feedback #85(u8 0) -> (w1971:u8)
            n982 = Add(x=w1970, y=w1971) -> (x+y=w1969:u8)
            "Blue Late Counter (D)" <- w1969
            n983 = feedback-in #85(w1969) -> ()
            n984 = Subtract(x=w1977, y=w1976) -> (x-y=w1975:i16)
            "BI Relative phase (D)" <- w1975
            n985 = feedback-in #84(w1975) -> ()
            n986 = feedback #86(TRUE) -> (w1984:bool)
            n987 = case shown="2" "Blue Laser Operating Mode (D)" {
              tunnel: [TRUE FALSE w1998] -> w1962
              tunnel: w1984 -> [_ _ w1995]
              frame 0, Default {
              }
              frame 1 {
              }
              frame 2 {
                n988 = Not(x=w1995) -> (.not. x?=w1997:bool)
                n989 = Select(t=w1997, s="Invert BI (D)", f=w1995) -> (s? t:f=w1998:bool)
              }
            }
            n990 = Subtract(x=w1957, y="Lifetime events to read blue") -> (x-y=w1955:u16)
            n991 = Not(x=w1984) -> (.not. x?=w1982:bool)
            n992 = Select(t="Blue interlace ON count (D)", s=w1982, f="Blue interlace OFF count (D)") -> (s? t:f=w1986:u16)
            n993 = Subtract(x=w1986, y=w1967) -> (x-y=w1980:u16)
            n994 = Add(x=w1980, y=w1976) -> (x+y=w1974:u16)
            n995 = feedback-in #86(w1982) -> ()
            n996 = Select(t=w1955, s="Lifetime read blue fifo", f=w1957) -> (s? t:f=w1958:u16)
            "lifetime events in fifo" <- w1958
            n997 = Equal?(x="Blue Laser Operating Mode (D)", y=u8 2) -> (x = y?=w1963:bool)
            n998 = Not(x=w1962) -> (.not. x?=w1961:bool)
            n999 = And(x=w1961, y=w1963) -> (x .and. y?=w1960:bool)
          }
        }
      }
    }
    frame Enabled {
    }
  }
